vi "main_ui.vi"() -> ()   [LabVIEW 2014]
uses:
  <vilib>/Utility/miscctls.llb/LVPointDoubleTypeDef.ctl
  <vilib>/Analysis/1siggen.llb/Ramp Pattern by Samples.vi
  src/GLOBAL_VAR.vi
  <vilib>/Analysis/NI_AALBase.lvlib
panel:
  out "Laser power [mW]":dbl caption="Power" format="%.3f"
  in  "laser_on-off":bool caption="Laser"
  in  "T1_open":bool caption="Open T1"
  in  "esr_start":bool caption="Open ESR"
  in  "stop":bool
  in  "scan_start":bool
  in  "live-scan":bool
  out "ESR_stack":dbl[][](graph)
  out "X":dbl caption="X Rel" format="%.3f"
  out "Y":dbl caption="Y Rel" format="%.3f"
  out "XY Graph 2":cluster{"Value":dbl[], "Ramp Pattern":dbl[]}(graph)={"Value"=[-75.0, -71.93877551020408, -68.87755102040816, -65.81632653061224, -62.755102040816325, -59.69387755102041, -56.63265306122449, -53.57142857142857, -50.51020408163265, -47.44897959183673, -44.38775510204081, -41.3265306122449, -38.26530612244898, -35.204081632653065, -32.142857142857146, -29.081632653061227, -26.02040816326531, -22.95918367346939, -19.89795918367347, -16.836734693877553, -13.775510204081634, -10.714285714285722, -7.653061224489804, -4.591836734693885, -1.5306122448979664, 1.5306122448979522, 4.591836734693871, 7.6530612244897895, 10.714285714285708, 13.775510204081627, 16.836734693877546, 19.897959183673464, 22.959183673469383, 26.0204081632653, 29.08163265306122, 32.14285714285714, 35.20408163265306, 38.265306122448976, 41.326530612244895, 44.38775510204081, 47.44897959183673, 50.51020408163265, 53.571428571428555, 56.63265306122449, 59.69387755102039, 62.755102040816325, 65.81632653061223, 68.87755102040816, 71.93877551020407, 75.0], "Ramp Pattern"=[0.0, 0.0, 0.0, 0.0, 0.0, 0.0, 0.0, 0.0, 0.0, 0.0, 0.0, 0.0, 0.0, 0.0, 0.0, 0.0, 0.0, 0.0, 0.0, 0.0, 0.0, 0.0, 0.0, 0.0, 0.0, 0.0, 0.0, 0.0, 0.0, 0.0, 0.0, 0.0, 0.0, 0.0, 0.0, 0.0, 0.0, 0.0, 0.0, 0.0, 0.0, 0.0, 0.0, 0.0, 0.0, 0.0, 0.0, 0.0, 0.0, 0.0]}
  out "XY Graph":cluster{"Value":dbl[], "Ramp Pattern":dbl[]}(graph)={"Value"=[0.0, 0.0, 0.0, 0.0, 0.0, 0.0, 0.0, 0.0, 0.0, 0.0, 0.0, 0.0, 0.0, 0.0, 0.0, 0.0, 0.0, 0.0, 0.0, 0.0, 0.0, 0.0, 0.0, 0.0, 0.0, 0.0, 0.0, 0.0, 0.0, 0.0, 0.0, 0.0, 0.0, 0.0, 0.0, 0.0, 0.0, 0.0, 0.0, 0.0, 0.0, 0.0, 0.0, 0.0, 0.0, 0.0, 0.0, 0.0, 0.0, 0.0], "Ramp Pattern"=[-75.0, -71.93877551020408, -68.87755102040816, -65.81632653061224, -62.755102040816325, -59.69387755102041, -56.63265306122449, -53.57142857142857, -50.51020408163265, -47.44897959183673, -44.38775510204081, -41.3265306122449, -38.26530612244898, -35.204081632653065, -32.142857142857146, -29.081632653061227, -26.02040816326531, -22.95918367346939, -19.89795918367347, -16.836734693877553, -13.775510204081634, -10.714285714285722, -7.653061224489804, -4.591836734693885, -1.5306122448979664, 1.5306122448979522, 4.591836734693871, 7.6530612244897895, 10.714285714285708, 13.775510204081627, 16.836734693877546, 19.897959183673464, 22.959183673469383, 26.0204081632653, 29.08163265306122, 32.14285714285714, 35.20408163265306, 38.265306122448976, 41.326530612244895, 44.38775510204081, 47.44897959183673, 50.51020408163265, 53.571428571428555, 56.63265306122449, 59.69387755102039, 62.755102040816325, 65.81632653061223, 68.87755102040816, 71.93877551020407, 75.0]}
  out "scan_image":dbl[][](graph)
  out "wavechart_01":dbl(graph)
  in  "Tab Control":T1(tab)
  in  "counting_start":bool
  out "counts":dbl format="%.3e"
  in  "counts_dwell_time":dbl=30.0 caption="Dwell time [ms] :" min=0.0
  in  "pos-zero":bool caption="Blank Button"
  in  "scan_direction":enum32{"0", "1"}(radio)=enum."1" caption="Scan direction:"
  in  "frame_size_x_px":i32=100 caption="image_size_x"
  out "frame_size_y_px":i32=100 caption="image_size_y"
  out "pixel_size_z_um":dbl format="%#_3g"
  out "pixel_size_x_um":dbl=1.5 format="%#_3g"
  out "pixel_size_y_um":dbl=1.5 format="%#_3g"
  in  "pixel_dwell_ms":dbl=1.0 caption="Dwell time:"
  out "time_frame_s":dbl=10.0 caption="Time per frame:"
  in  "cursor-reset":bool caption="Blank Button"
  in  "pos-start_y":dbl caption="Y:" format="%#.3g"
  in  "pos-start_x":dbl caption="X:" format="%#.3f"
  in  "pos-start_cursor":bool caption="Blank Button"
  in  "pos_start":enum32{"bottom-left", "center"}(radio)=enum."center"
  in  "image_size_x_um":dbl=150.0 caption="X:"
  out "image_size_y_um":dbl=150.0 caption="Y:"
  in  "pos_z":dbl(slide) caption="Z:" scale=45.0..55.0
  in  "focus_z":dbl caption="Focus :" min=0.0 max=100.0 step=0.001 format="%.3f"
  in  "focus_dwell_ms":dbl=100.0 caption="Dwell :"
  in  "focus_q_steps":i32=100 caption="Steps :"
  in  "focus_z_end":dbl=100.0 caption="End :"
  in  "focus_z_start":dbl caption="Start :"
  in  "focus_start":bool
  out "timeseries-rem_time":string caption="Remaining time :"
  in  "timeseries-autofocus":enum16{"No autofocus", "Max x-y", "Center"}(ring) caption="Autofocus :"
  out "timeseries-current_image":dbl caption="Current scan :" format="%#.3f"
  out "timeseries-total_images":dbl=1.0 caption="Total scans :" format="%#.3f"
  in  "timeseries-start":bool
  in  "timeseries-period":dbl caption="Period :" format="%#.3f"
  in  "timeseries-stopdate":timestamp=timestamp(3557915984.536238 s since 1904-01-01) caption="Stop at :" format="%<%X\n%x>T"
  out "timeseries-next_scan":timestamp caption="Next scan at :" format="%<%X\n%x>T"
  in  "Z-stack_enable":bool
  in  "z-stack_slices":i32=1 caption="Slices :" min=1 step=1
  out "z-stack_step_size":dbl caption="Step size :" format="%#.4f"
  in  "Z-stack_tabs":enum32{"From-To", "Centering"}(tab)
  in  "z-stack-set_to":bool
  in  "z-stack-set_from":bool
  in  "z-stack_to":dbl=100.0 caption="To :"
  in  "z-stack_from":dbl caption="From :"
  in  "z-stack-set_center":bool
  in  "z-stack_size":dbl=10.0 caption="Size :"
  in  "z-stack_center":dbl=5.0 caption="Center :"
  in  "z-stack_pos":i32(slide)=1 caption="Z slice :" min=1 step=1 scale=1.0..1.1
  in  "current_z":dbl caption="Z :" min=0.0 max=100.0 step=0.0001 format="%.4f"
  in  "current_y":dbl caption="Y :" min=-10.0 max=10.0 step=0.0001 format="%.4f"
  in  "current_x":dbl caption="X :" min=-10.0 max=10.0 step=0.0001 format="%.4f"
  in  "recenter":bool caption="Laser"
  in  "continious_recenter":bool
  in  "parameters_xy-scan":T2={"image_size_xy_um"=0.5, "frame_size_xy_px"=20, "dwell_time_ms"=1.0}
  in  "parameters_z-scan":T3={"dwell_time_ms"=10.0, "q_steps"=20, "span_um"=2.0, "refocus"=TRUE}
  out "particle_lost":bool
  in  "XY Max focus?":bool
  in  "X Zero":dbl format="%.3f"
  in  "Y Zero":dbl format="%.3f"
  in  "X Rel":dbl format="%.3f"
  in  "Y Rel":dbl format="%.3f"
  out "upos-xy_control":cluster{"X":dbl, "Y":dbl}[](graph)
  in  "upos-stop":bool
  in  "upos-x":dbl caption="X:" min=0.0 max=8.0 format="%.3f"
  in  "upos-y":dbl caption="Y:" min=0.0 max=8.0 format="%.3f"
  out "upos-cpos_y":dbl format="%#.3f"
  out "upos-cpos_x":dbl format="%#.3f"
  out "upos-state_x":u32 caption="X:"
  out "upos-state_y":u32 caption="Y:"
  in  "tiles-overlap":dbl=10.0 caption="Overlap :"
  out "tile_progress":u8(slide) caption="Progress :" scale=0.0..100.0
  out "tile_remaining_tiles":dbl caption="Remaining\ntiles :"
  out "tile_remaining_time":dbl caption="Remaining\ntime :"
  in  "tile-scan_start":bool
  in  "tile_tiles-size":enum32{"tiles", "size"}(radio)=enum."size"
  out "tile_q-tiles_y":dbl=1.0 caption="Y :"
  in  "tile_q-tiles_x":dbl=1.0 caption="X :"
  out "tile_size_y_um":dbl=10.0 caption="Y:"
  in  "tile_size_x_um":dbl=10.0 caption="Size :"
  in  "tile_start_y_mm":dbl caption="Y:" format="%#.3g"
  in  "tile_start_x_mm":dbl caption="X:" format="%#.3f"
  out "esr_generator_ok":bool caption="Generator\nstatus :"
  out "esr_current_run":i32 caption="Run :"
  in  "esr_out_enable":bool caption="Output on/off :"
  out "esr_power_led":bool
  out "esr_remain":i32 caption="Remain :"
  in  "esr_repetitions":i32=1 caption="Repetitions" min=1 max=1000 step=1
  in  "esr_dwell_time":ext=0.09999999974525053 caption="Dwell Time :" format="%.3f"
  in  "esr_step_size":ext=2500000.0 caption="Step size :" format="%.2p"
  in  "esr_freq_stop":ext=3000000000.0 caption="Freq Stop :" format="%.2p"
  in  "esr_freq_start":ext=2800000000.0 caption="Freq Start :" format="%.2p"
  out "esr_total_time":ext=8120.249980327117 caption="Total time :"
  in  "esr_power":ext=5.999999061226845 caption="Power :" format="%.2f"
  in  "live_scan_direction":enum32{"0", "1"}(radio)=enum."1" caption="Scan direction:"
  in  "live_frame_size_x_px":i32=50 caption="image_size_x"
  in  "live_pixel_dwell_ms":dbl=0.5 caption="Dwell time:"
  in  "objective":u16(ring)=1 items=["Raw scale (volts)", "UPlanSApo 100x / 1,40 Oil", "UPlanSApo 40X / 0,95 Air"]
  in  "file_save":bool
  in  "file_autosave":bool
  in  "file_path":path caption="Folder :"
  in  "file_name":string caption="Name :"
  in  "save_tiff":bool
  in  "save_txt":bool
  # "Relative cursor position [um]"
  # "Scanning area [mm]"
  # "Size:"
  # "x"
  # "Position:"
  # "Acquisition"
  # "Frame size:"
  # "x"
  # "px"
  # "ms"
  # "Pixel size [mm] :"
  # "x"
  # "x"
  # "Seconds"
  # "Manual focus [mm]"
  # "Auto-focus [mm]"
  # "ms"
  # "Photon counting"
  # "Time series"
  # "[s]"
  # "Z stack [mm]"
  # "Set position [mm]"
  # "Refocus"
  # "Positioners (xy motors)"
  # "Absolute"
  # "Zeros"
  # "Relative"
  # "Status"
  # "State :"
  # "Position :"
  # "Tiles scan"
  # "Start position [mm]:"
  # "mm"
  # "mm"
  # "mm"
  # "min"
  # "Sweep"
  # "Hz"
  # "Hz"
  # "Hz"
  # "ms"
  # "dBm"
  # "s"
  # "Objective"
  # "Live scan"
  # "Frame size:"
  # "px"
  # "ms"
  # "Save"
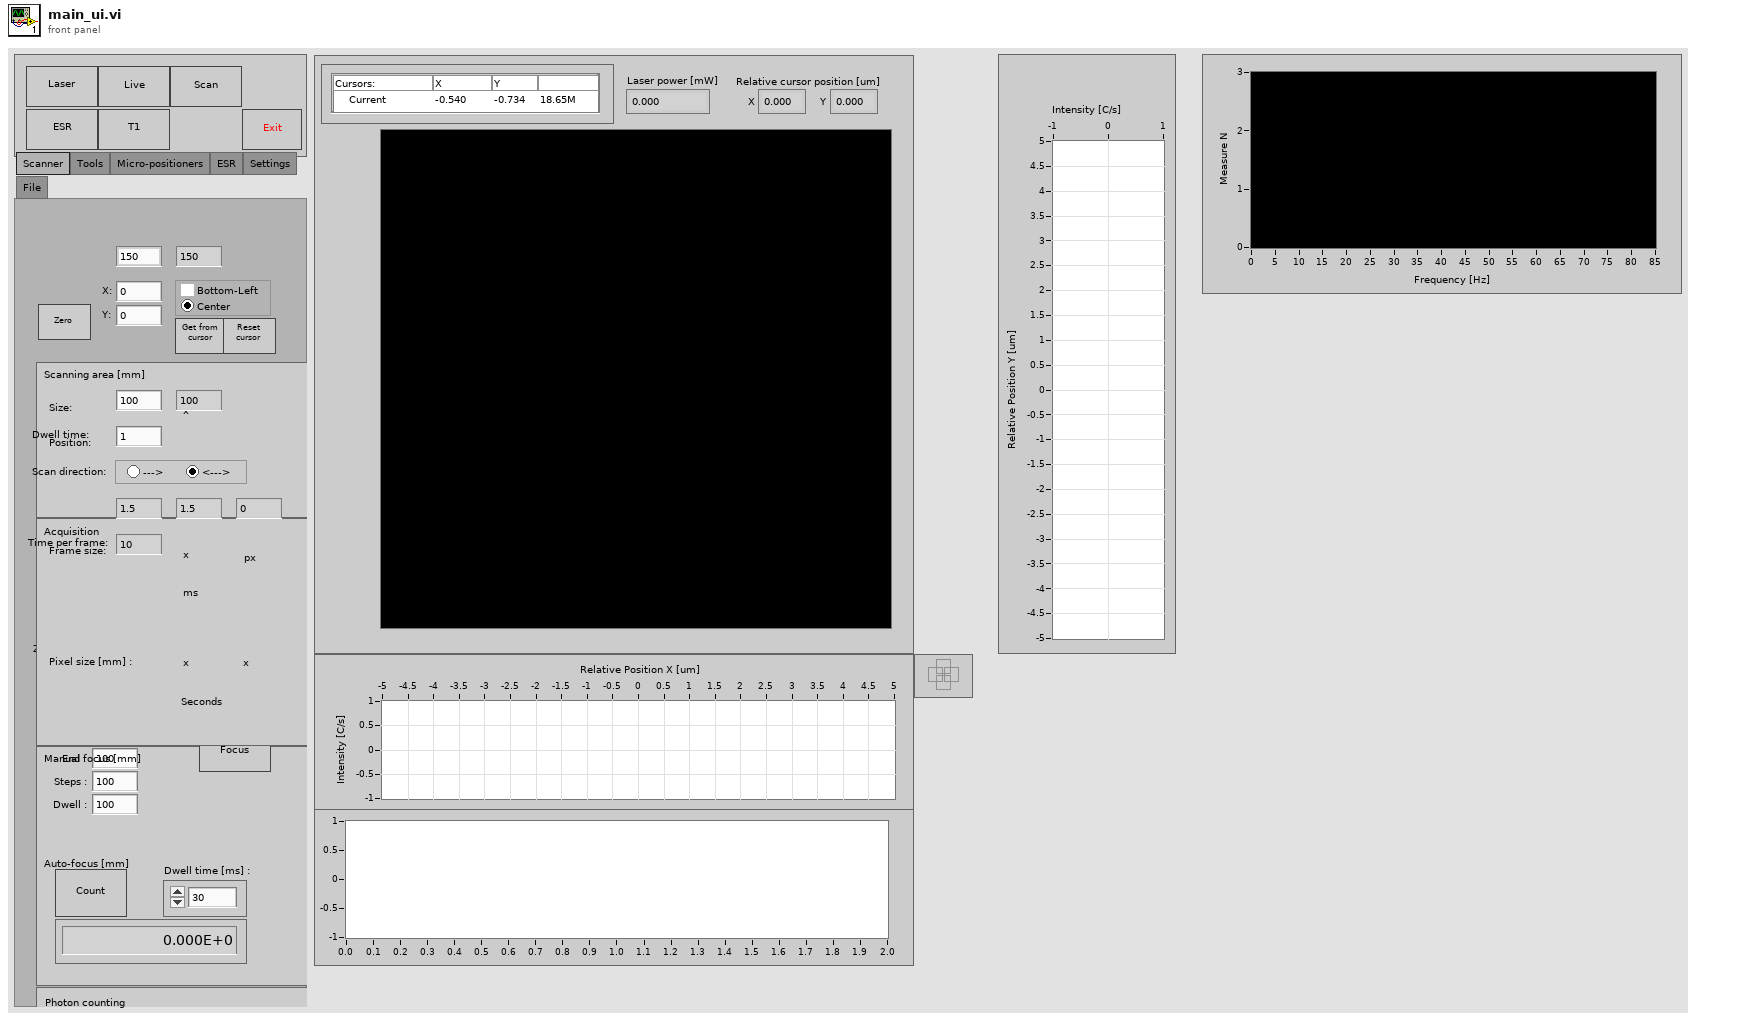
[diagram p1: front panel]
types:
  T1 = enum32{"Scanner", "Tools", "Micro-positioners", "ESR", "Settings", "File"}
  T2 = cluster{"image_size_xy_um":dbl, "frame_size_xy_px":u32, "dwell_time_ms":dbl}
  T3 = cluster{"dwell_time_ms":dbl, "q_steps":u32, "span_um":dbl, "refocus":bool}
  T4 = cluster{"status_x":dbl, "status_y":dbl, "status_z":dbl, "pos_x":dbl, "pos_y":dbl, "pos_z":dbl}
  T5 = cluster{enum16{"standby", "domove", "dostop", "exit", "status"}, dbl, dbl, dbl}
  T6 = typedef "LVPointDoubleTypeDef.ctl" = cluster{"X":dbl, "Y":dbl}
  T7 = enum8{"Enabled", "Disabled", "Disabled and Grayed Out"}
  T8 = cluster{"overlap":dbl, "pos-xy_start":cluster{"pos-x_start":dbl, "pos-y_start":dbl}, "pos-xy_end":cluster{"pos-x_end":dbl, "pos-y_end":dbl}, "pos-xy_ref":cluster{"pos-x_start":dbl, "pos-y_start":dbl}}
  T9 = cluster{"z_start":dbl, "z_end":dbl, "q_steps":i32, "dwell_time_ms":dbl}
  T10 = cluster{"image_size":dbl, "image_xy_start":cluster{"image-x_start":dbl, "image-y_start":dbl}, "pixel_dwell_ms":dbl, "frame_size_x_px":i32, "scan_direction":enum32{"0", "1"}, "pos_start":enum32{"bottom-left", "center"}}
  T11 = cluster{"nano-position_X_um":sgl, "nano-position_Y_um":sgl, "nano-position Z_um":sgl}
  T12 = enum16{"Standby", "doScan", "doCount", "doFocus", "doLiveScan", "do3DScan"}
  T13 = enum16{"Standby", "doScan", "doCount", "doFocus", "doLiveScan"}
  T14 = enum16{"Standby", "doScan", "doCount", "doFocus", "doLiveScan", "do3DScan", "changeZslice", "doESR", "doTileScan", "doStartPos", "doTimeseries"}
  T15 = enum16{"Standby", "doScan", "doCount", "doFocus"}
  T16 = enum16{"Standby", "doScan", "doCount", "doFocus", "doLiveScan", "do3DScan", "changeZslice", "doESR", "doTileScan", "doStartPos", "doTimeseries", "saveImage", "doT1", "doRecenter"}
  T17 = enum16{"Standby", "doScan", "doCount", "doFocus", "doLiveScan", "do3DScan", "changeZslice"}
  T18 = enum16{"Standby", "doScan", "doCount", "doFocus", "doLiveScan", "do3DScan", "changeZslice", "doESR"}
  T19 = enum16{"Standby", "doScan", "doCount", "doFocus", "doLiveScan", "do3DScan", "changeZslice", "doESR", "doTileScan"}
  T20 = enum16{"standby", "domove", "dostop", "exit", "status"}
  T21 = enum16{"Standby", "doScan", "doCount", "doFocus", "doLiveScan", "do3DScan", "changeZslice", "doESR", "doTileScan", "doStartPos", "doTimeseries", "saveImage", "doT1"}
  T22 = enum16{"Standby", "doScan", "doCount", "doFocus", "doLiveScan", "do3DScan", "changeZslice", "doESR", "doTileScan", "doStartPos", "doTimeseries", "saveImage"}
  T23 = cluster{enum16{"standby", "domove", "dostop", "exit", "status"}, "Value":dbl, "Value":dbl, "Value":dbl}
  T24 = cluster{enum16{"standby", "domove", "dostop", "exit", "status"}, dbl, dbl, "Value":dbl}
  T25 = cluster{enum16{"standby", "domove", "dostop"}, "X":dbl, "Y":dbl, dbl}
  T26 = cluster{enum16{"standby", "domove", "dostop", "exit"}, "upos-x":dbl, "upos-y":dbl, dbl}
  T27 = cluster{enum16{"standby", "domove", "dostop", "exit"}, dbl, dbl, dbl}
  T28 = cluster{"pos-start_x":dbl, "pos-start_y":dbl, "focus_z":dbl}
  T29 = cluster{"file_path":path, "file_name":string, "image":dbl[][][], "image_size_xy":cluster{"image_size_x_um":sgl, "image_size_y_um":sgl}, "pixel_dwell_time_ms":sgl, "Laser_power_mW":sgl, "pixel_size":dbl, "tile_ij":cluster{"tile_i":i32, "tile_j":i32}, "Objective":string, "ColorMarkers":cluster{dbl, u32}[], "timestamp":timestamp, "micro-position-xyz":cluster{"micro-position_x_mm":sgl, "micro-position_y_mm":sgl, "micro-position_z_mm":sgl}, "zero_xyz":cluster{"zero_x_mm":dbl, "zero_y_mm":dbl, "zero_z_mm":dbl}, "nano-position-xyz":cluster{"nano-position_x_V":sgl, "nano-position_y_V":sgl, "nano-position_z_V":sgl}, "Kxyz":cluster{"Kx_V/um":sgl, "Ky_V/um":sgl, "Kz_V/um":sgl}}
  T30 = cluster{"image_size_x_um":dbl, "image_size_x_um":dbl}
  T31 = cluster{"esr_repetitions":i32, "esr_power":ext, "esr_freq_start":ext, "esr_freq_stop":ext, "esr_step_size":ext, "esr_dwell_time":ext}
  T32 = cluster{"Cursor.Cursor X":dbl, "Cursor.Cursor Y":dbl, "focus_z":dbl}
  T33 = cluster{"tile_start_x_mm":dbl, "tile_start_y_mm":dbl}
  T34 = cluster{"Value":dbl, "Value":dbl, "Value":i32, "Value":bool}
  T35 = cluster{"timeseries-current_image":refnum<vi>, "scan_image":refnum<vi>, "timeseries-start":refnum<vi>, "timeseries-next_scan":refnum<vi>, "timeseries-rem_time":refnum<vi>}
  T36 = cluster{"X Zero":dbl, "Y Zero":dbl, "upos-y":dbl}
  T37 = cluster{"Cursor.Cursor X":dbl, "Cursor.Cursor Y":dbl, "Value":dbl}
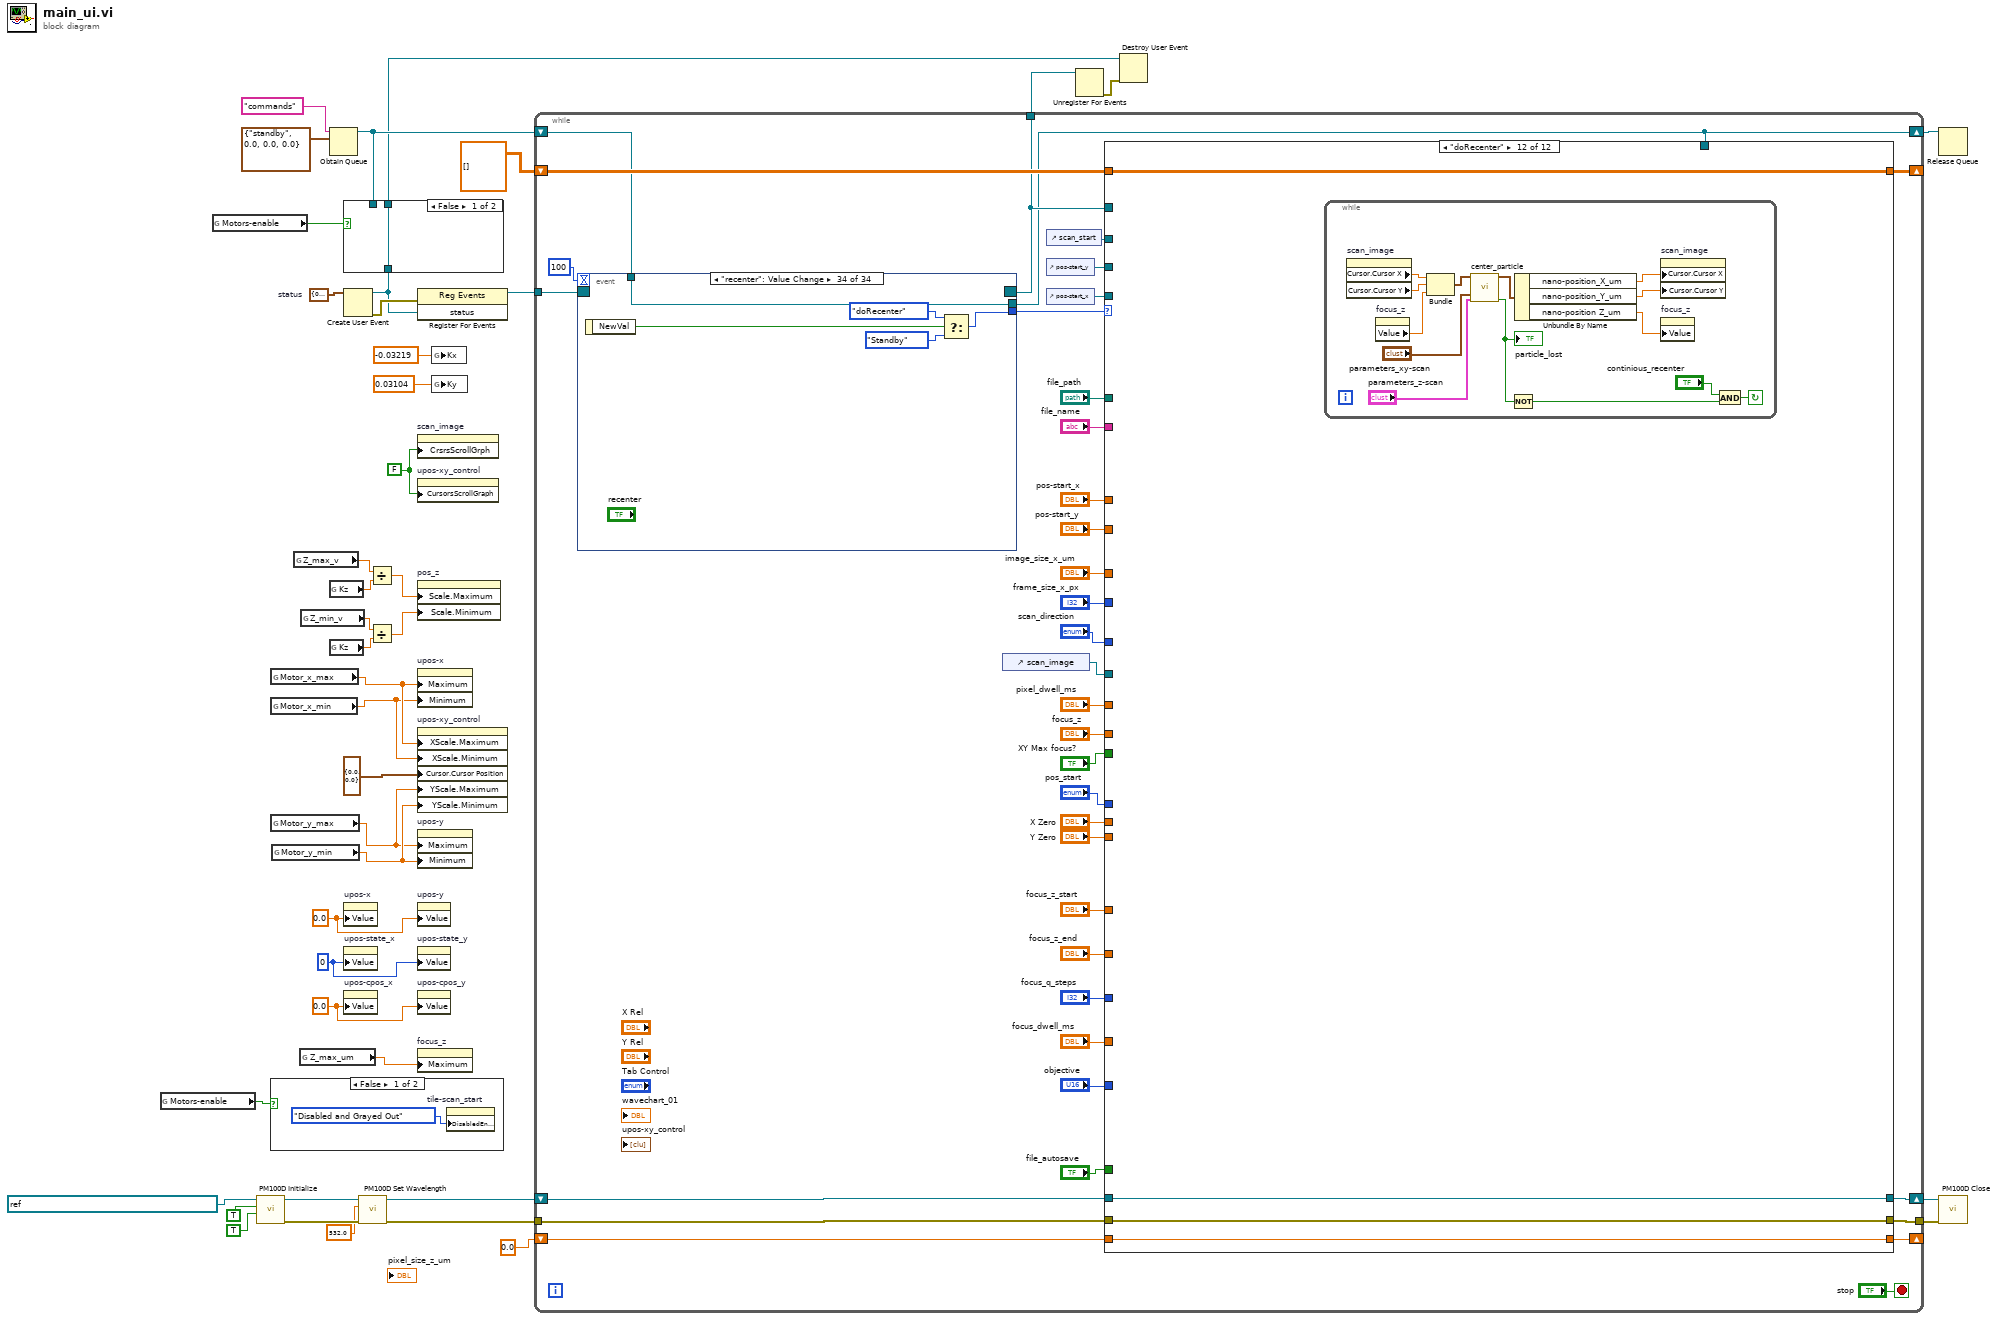
[diagram p0: block diagram]
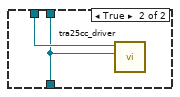
[diagram p2: hidden frame]
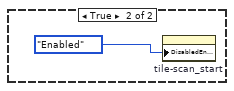
[diagram p3: hidden frame]
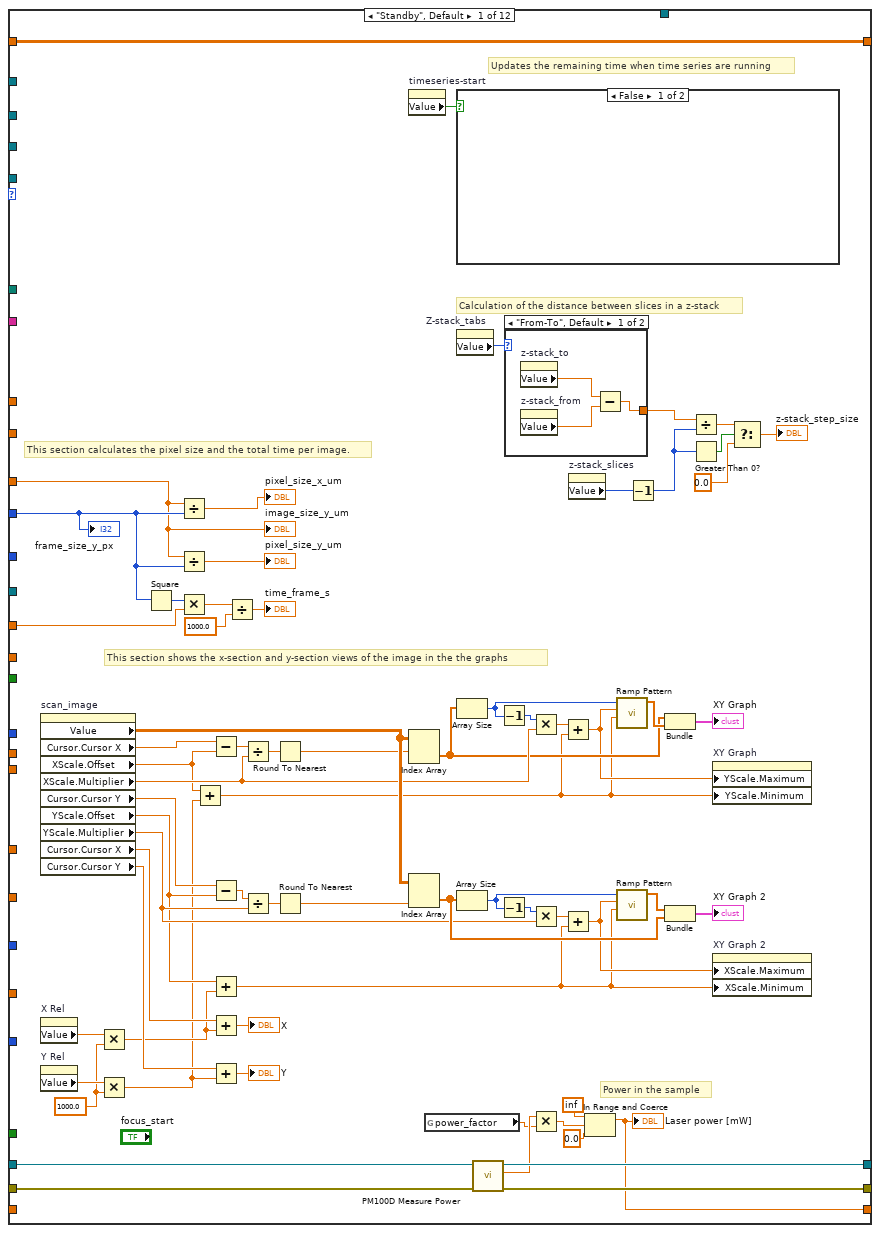
[diagram p4: hidden frame]
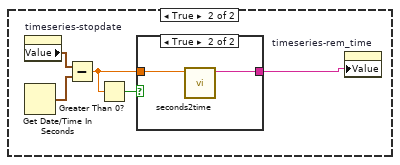
[diagram p5: hidden frame]
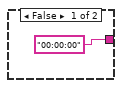
[diagram p6: hidden frame]
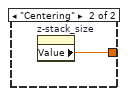
[diagram p7: hidden frame]
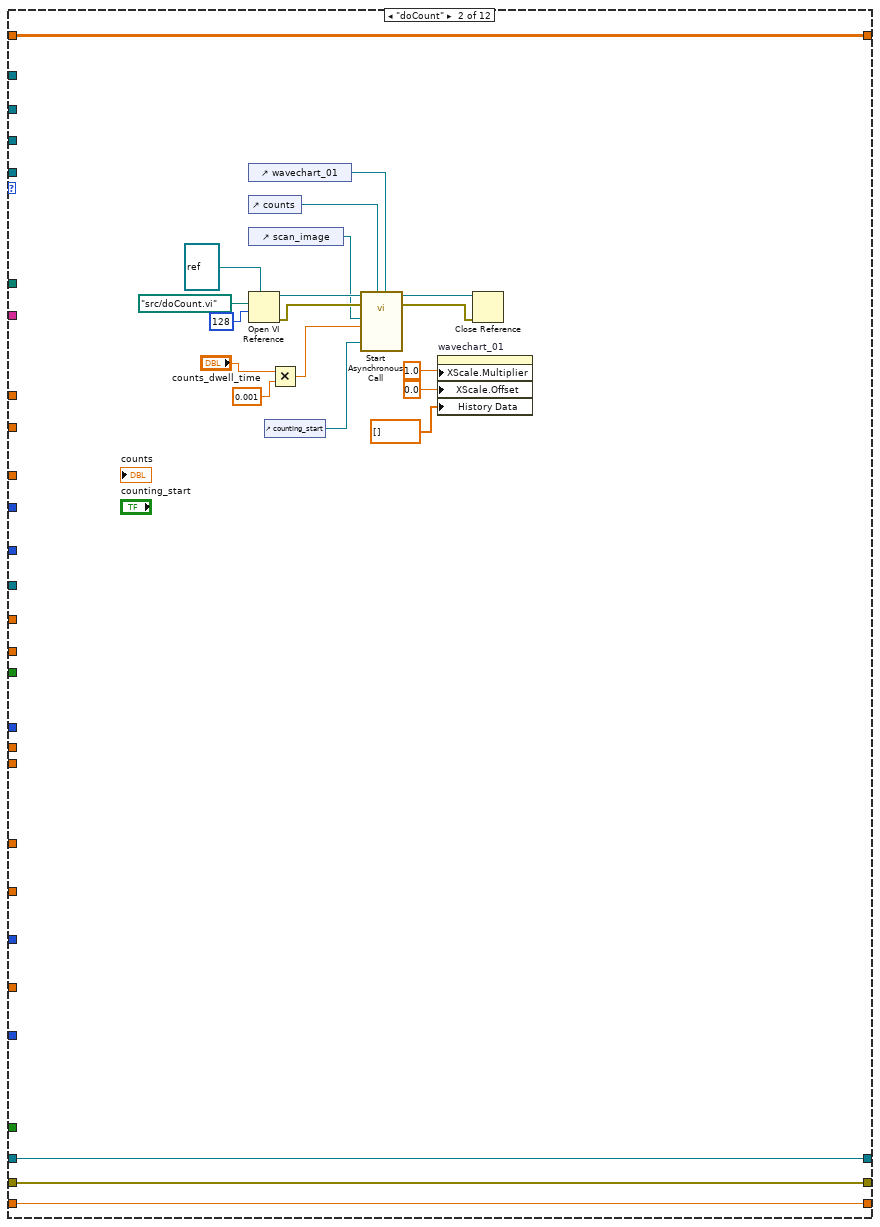
[diagram p8: hidden frame]
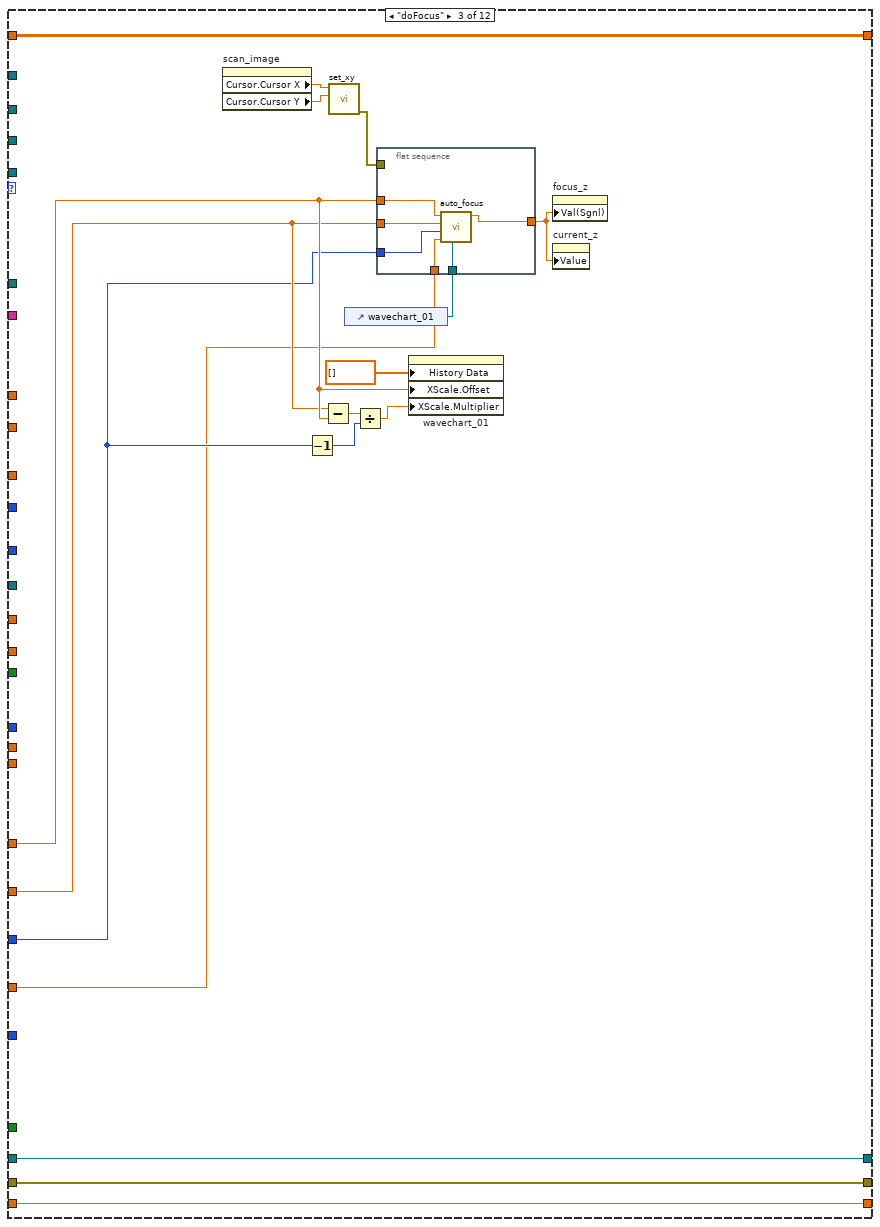
[diagram p9: hidden frame]
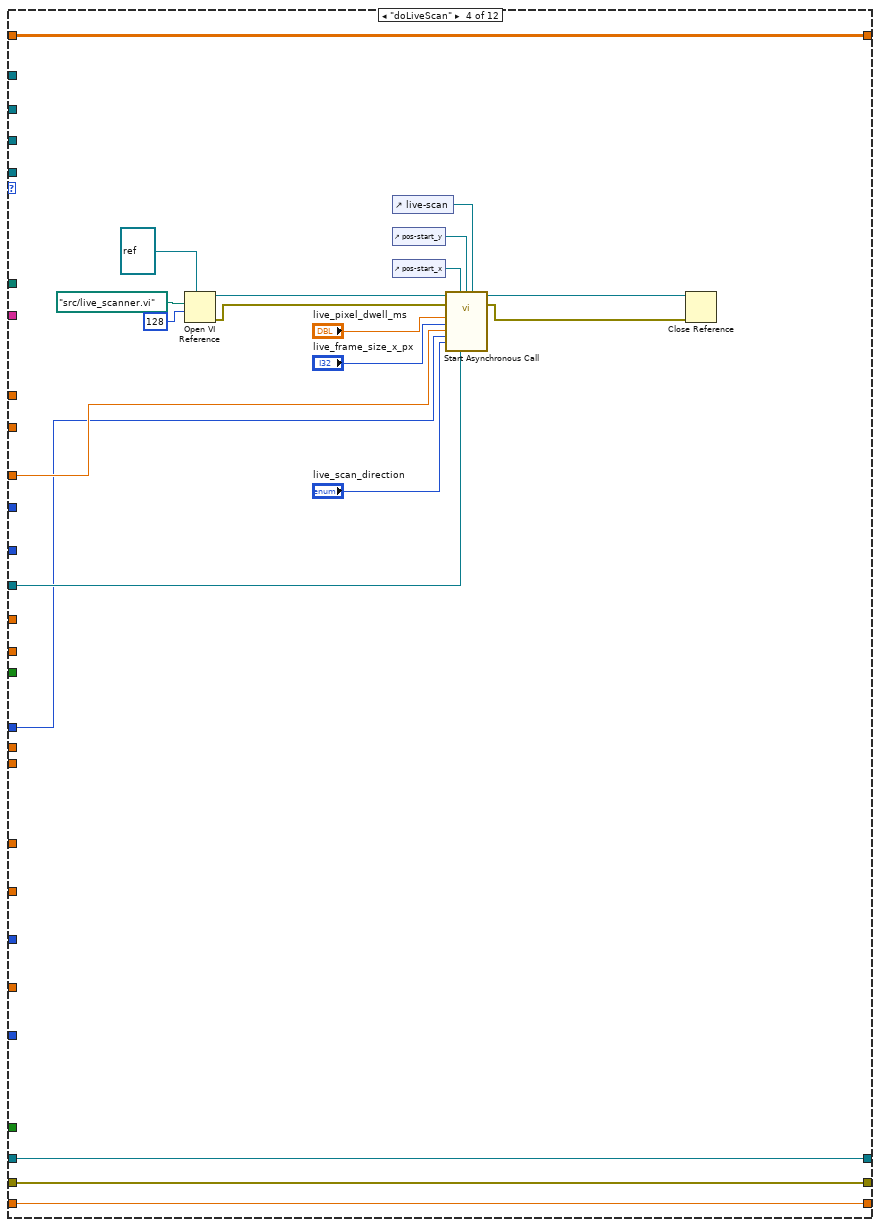
[diagram p10: hidden frame]
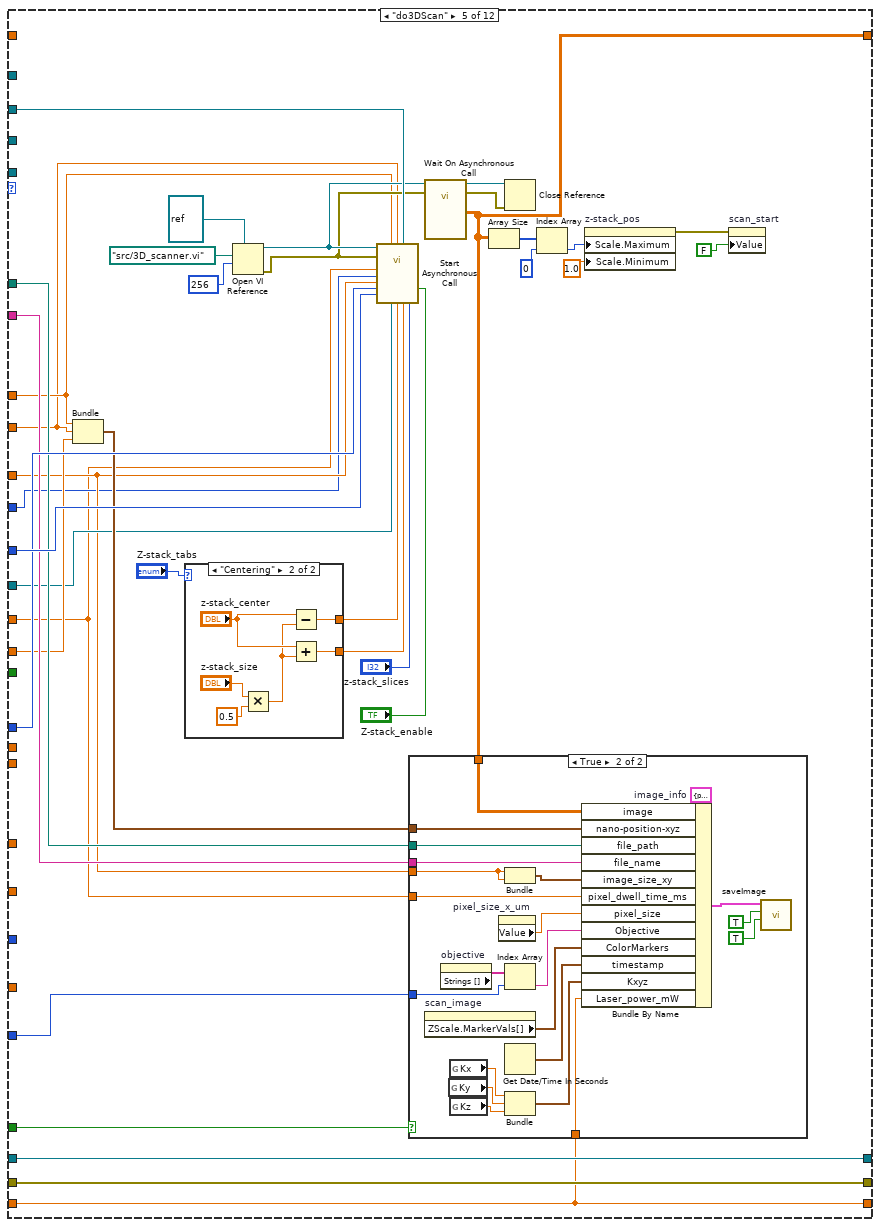
[diagram p11: hidden frame]
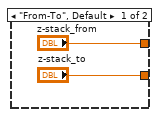
[diagram p13: hidden frame]
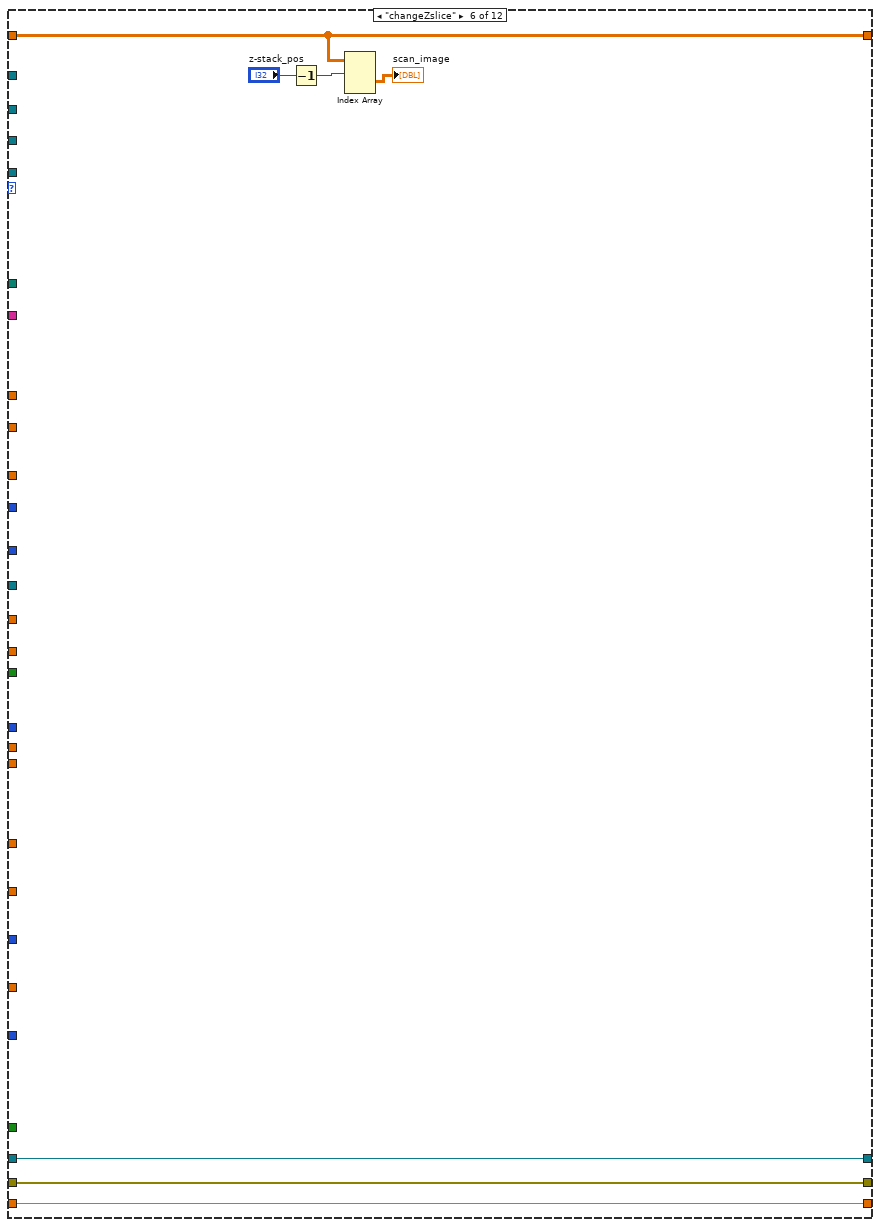
[diagram p14: hidden frame]
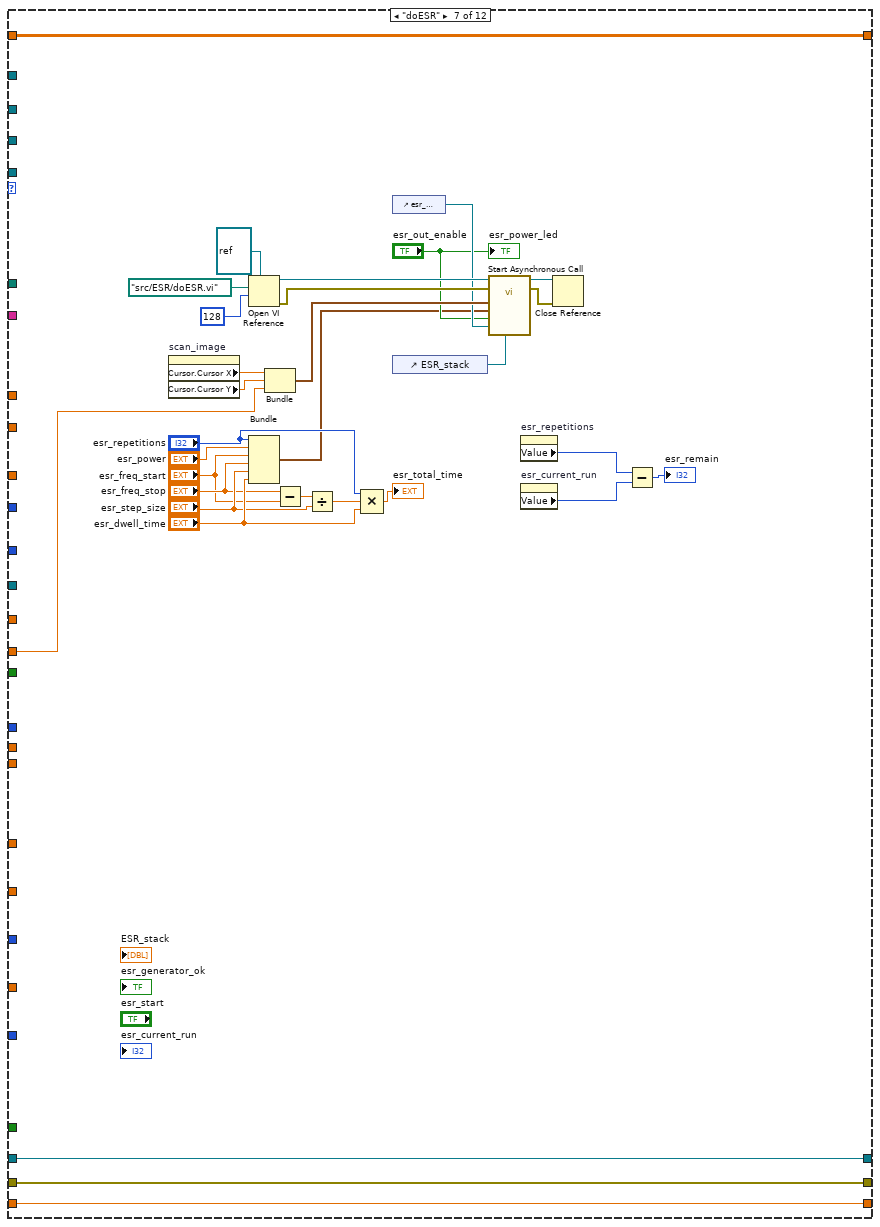
[diagram p15: hidden frame]
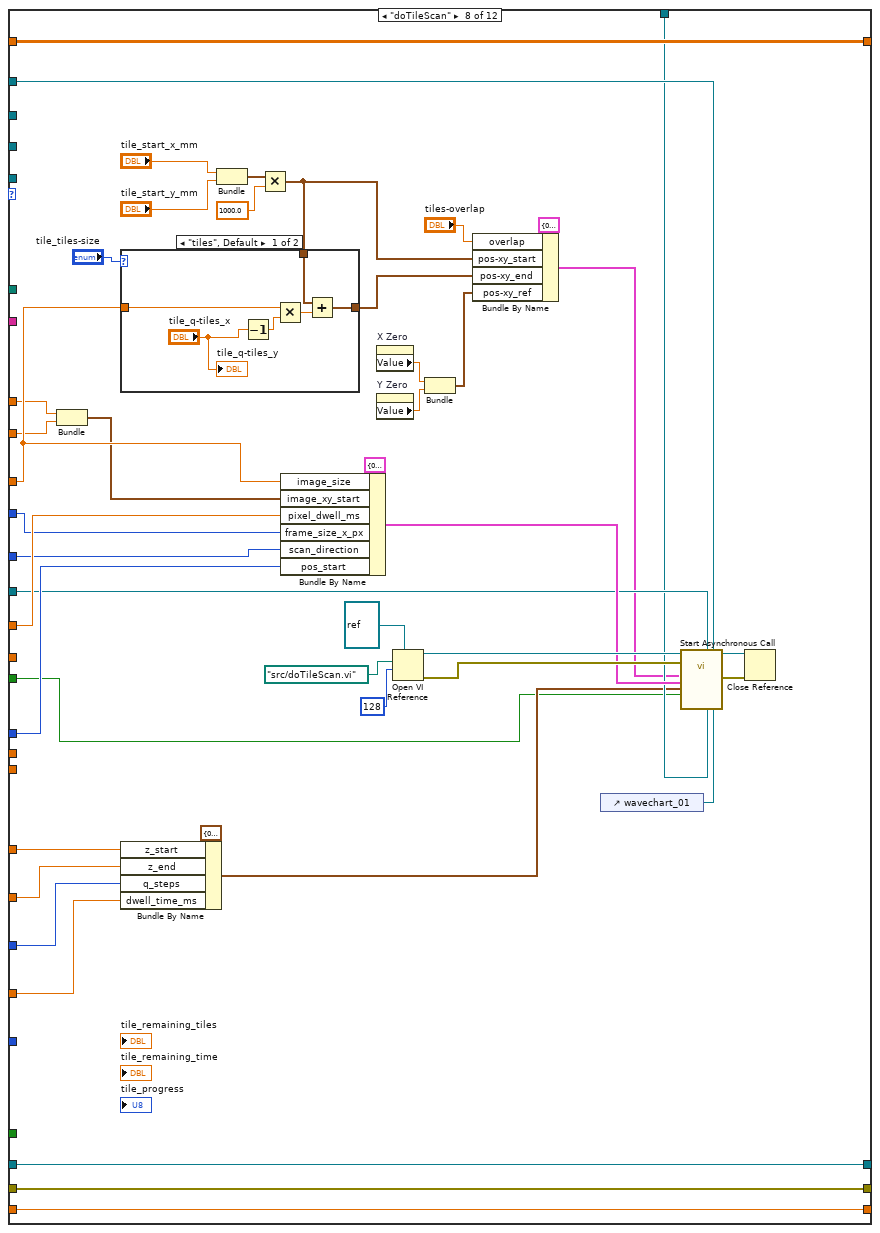
[diagram p16: hidden frame]
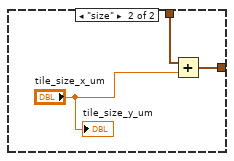
[diagram p17: hidden frame]
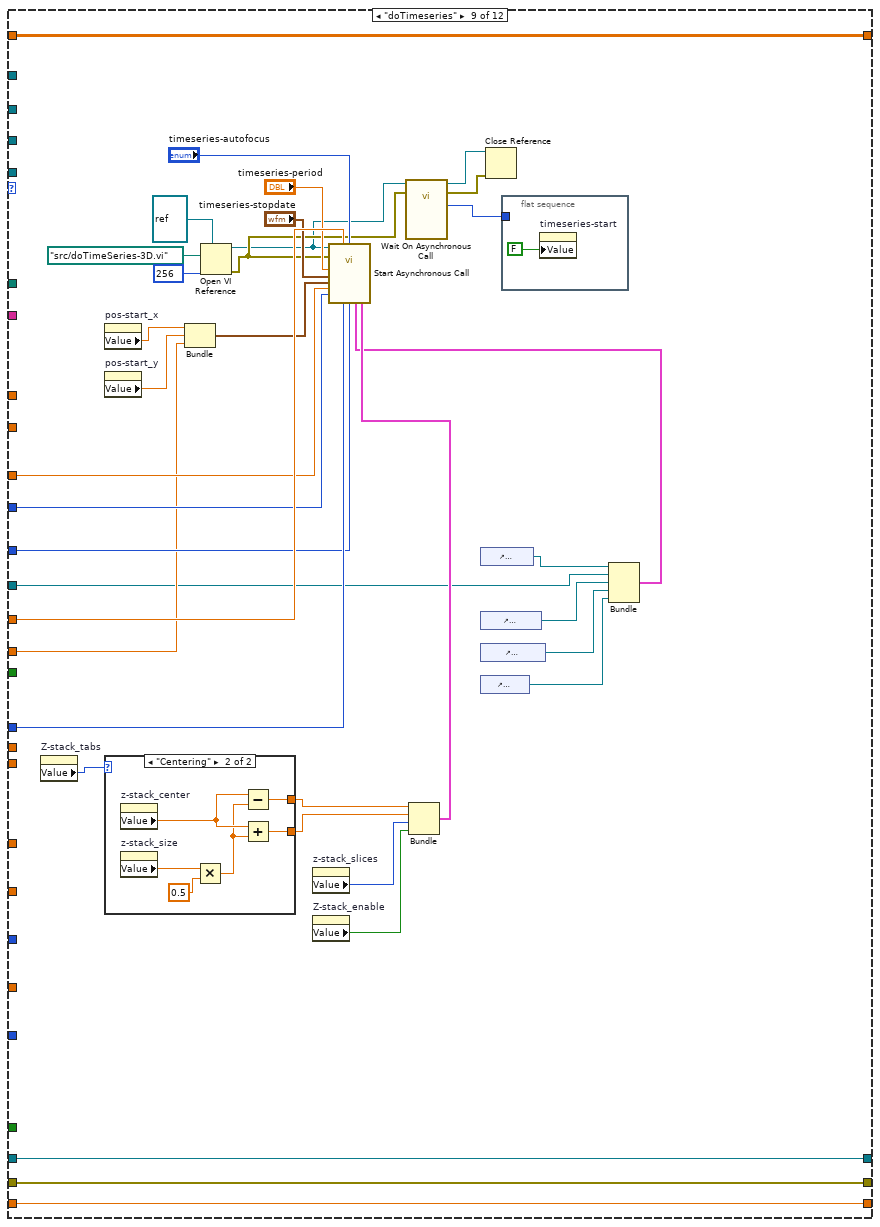
[diagram p18: hidden frame]
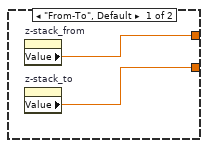
[diagram p19: hidden frame]
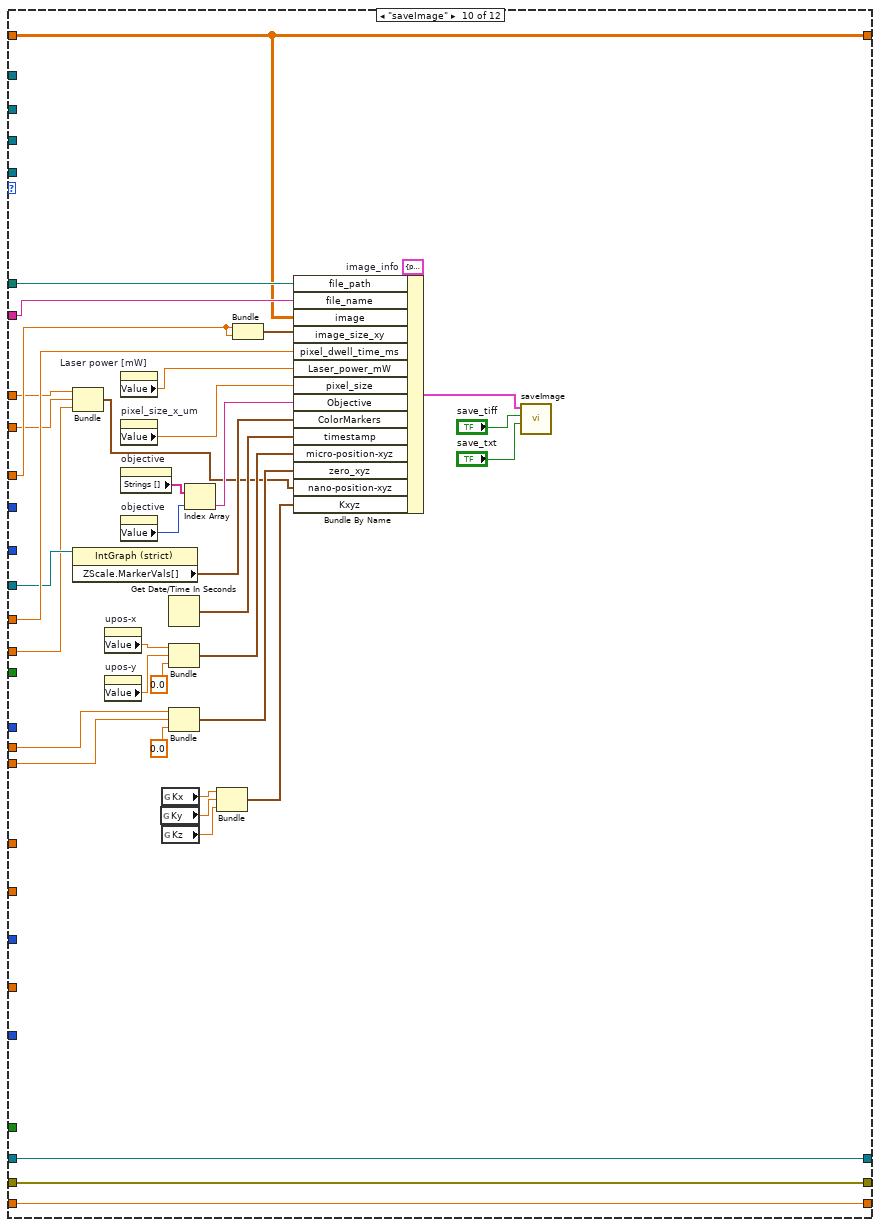
[diagram p20: hidden frame]
diagram:
  w24 = T4 {"status_x"=0.0, "status_y"=0.0, "status_z"=0.0, "pos_x"=0.0, "pos_y"=0.0, "pos_z"=0.0}  # status
  w28 = 0.0 ("upos-cpos_x")
  w29 = u32 0 ("upos-state_x")
  w30 = 0.0 ("upos-x")
  w36 = FALSE ("Cursors Scroll Graph")
  n1 = global read "GLOBAL_VAR.vi" "Motors-enable"() -> (w27:bool)
  n2 = global read "GLOBAL_VAR.vi" "Motors-enable"() -> (w17:bool)
  n3 = call <instrlib>:"PM100D Initialize.vi"("Reset Device (Reset Device)"=TRUE ("ID Query (Do Query)"), "ID Query (Do Query)"=TRUE, "resource name"=refnum<visa-resource-name> "USB0::0x1313::0x8072::P2008372::INSTR") -> ("error out"=w5:errorcluster, "instrument handle out"=w4:refnum<visa-resource-name>)  [unwired: 7 in]
  n4 = global read "GLOBAL_VAR.vi" "Motor_x_max"() -> (w35:dbl)
  n5 = global read "GLOBAL_VAR.vi" "Motor_x_min"() -> (w34:dbl)
  n6 = global read "GLOBAL_VAR.vi" "Motor_y_max"() -> (w32:dbl)
  n7 = case shown="False" w27 {
    frame False {
      n8 = property on="tile-scan_start" class="Bool (strict)"("DisabledEnum"=T7."Disabled and Grayed Out" ("Disabled")) -> ()  [unwired: 2 in, 2 out]
    }
    frame True {
      n9 = property on="tile-scan_start" class="Bool (strict)"("DisabledEnum"=T7."Enabled" ("Disabled")) -> ()  [unwired: 2 in, 2 out]
    }
  }
  n10 = global read "GLOBAL_VAR.vi" "Motor_y_min"() -> (w33:dbl)
  n11 = global read "GLOBAL_VAR.vi" "Z_max_v"() -> (w43:dbl)
  n12 = global read "GLOBAL_VAR.vi" "Z_max_um"() -> (w12:dbl)
  n13 = global read "GLOBAL_VAR.vi" "Z_min_v"() -> (w40:dbl)
  n14 = Obtain Queue(name (unnamed)="commands", element data type=T5 {enum."standby", 0.0, 0.0, 0.0}) -> (queue out=w18:refnum<queue>)  [unwired: 3 in, 2 out]
  n15 = global read "GLOBAL_VAR.vi" "Kz"() -> (w42:dbl)
  n16 = global read "GLOBAL_VAR.vi" "Kz"() -> (w39:dbl)
  n17 = Create User Event(user event datatype=w24) -> (user event=w16:refnum<user-event>, error out=w23:errorcluster)  [unwired: 1 in]
  n18 = case shown="False" w17 {
    tunnel: w16 -> [w46 w47]
    tunnel: w18 -> [_ w48]
    tunnel: [w46 w47] -> w15
    frame False {
    }
    frame True {
      n19 = call "tra25cc_driver.vi"("user_event-status_in"=w47, "queue-commands"=w48) -> ()  [unwired: 9 in, 1 out]
    }
  }
  n20 = property on="upos-x" class="DigNum (strict)"("Value"=w30) -> ()  [unwired: 2 in, 2 out]
  n21 = property on="upos-state_x" class="DigNum (strict)"("Value"=w29) -> ()  [unwired: 2 in, 2 out]
  n22 = property on="upos-cpos_x" class="DigNum (strict)"("Value"=w28) -> ()  [unwired: 2 in, 2 out]
  n23 = call <instrlib>:"PM100D Set Wavelength.vi"("error in (no error)"=w5, "Wavelength (0.0)"=532.0, "instrument handle"=w4) -> ("error out"=w10:errorcluster, "instrument handle out"=w11:refnum<visa-resource-name>)  [unwired: 7 in]
  n24 = Divide(x=w43, y=w42) -> (x/y=w41:dbl)
  n25 = Divide(x=w40, y=w39) -> (x/y=w38:dbl)
  n26 = register-events(error in=w23, w16) -> (reference out=w22:refnum<event-registration>)  [unwired: 1 in, 1 out]
  n27 = property on="scan_image" class="IntGraph (strict)"("CrsrsScrollGrph"=w36) -> ()  [unwired: 2 in, 2 out]
  n28 = property on="upos-xy_control" class="XYGraph (strict)"("CursorsScrollGraph"=w36) -> ()  [unwired: 2 in, 2 out]
  n29 = property on="pos_z" class="Slide (strict)"("Scale.Maximum"=w41, "Scale.Minimum"=w38) -> ()  [unwired: 2 in, 2 out]
  n30 = property on="upos-x" class="DigNum (strict)"("Maximum"=w35, "Minimum"=w34) -> ()  [unwired: 2 in, 2 out]
  n31 = property on="upos-xy_control" class="XYGraph (strict)"("XScale.Maximum"=w35, "XScale.Minimum"=w34, "Cursor.Cursor Position"=T6 {"X"=0.0, "Y"=0.0}, "YScale.Maximum"=w32, "YScale.Minimum"=w33) -> ()  [unwired: 2 in, 2 out]
  n32 = property on="upos-y" class="DigNum (strict)"("Maximum"=w32, "Minimum"=w33) -> ()  [unwired: 2 in, 2 out]
  n33 = property on="upos-y" class="DigNum (strict)"("Value"=w30) -> ()  [unwired: 2 in, 2 out]
  n34 = property on="upos-state_y" class="DigNum (strict)"("Value"=w29) -> ()  [unwired: 2 in, 2 out]
  n35 = property on="upos-cpos_y" class="DigNum (strict)"("Value"=w28) -> ()  [unwired: 2 in, 2 out]
  n36 = property on="focus_z" class="DigNum (strict)"("Maximum"=w12) -> ()  [unwired: 2 in, 2 out]
  n37 = global write "GLOBAL_VAR.vi" "Kx"(-0.03219 ("Kx")) -> ()
  n38 = global write "GLOBAL_VAR.vi" "Ky"(0.03104 ("Kx")) -> ()
  n39 = while {
    shift-right: [w85] -> _
    shift-left: dbl[][][] [] ("image_out") -> [w84]
    tunnel: w22 -> [w74]
    tunnel: [w71] -> w21
    shift-right: [w70] -> w19
    shift-left: w18 -> [w72]
    tunnel: w10 -> [w61]
    tunnel: [w59] -> w9
    shift-right: [w52] -> _
    shift-left: 0.0 ("upper limit") -> [w51]
    shift-right: [w60] -> w8
    shift-left: w11 -> [w62]
    stop <- "stop" stop-if-true
    n40 = event shown="[33] \"recenter\": Value Change" {
      selector: w74 -> [_ _ _ _ _ _ _ _ _ _ _ _ _ _ _ _ _ _ _ _ _ _ _ _ _ _ _ _ _ _ _ _ _ _]
      dyn-events: [_ _ _ _ _ _ _ _ _ _ _ _ _ _ _ _ _ _ _ _ _ _ _ _ _ _ _ _ _ _ _ _ _ _] -> w71
      timeout: 100 -> [_ _ _ _ _ _ _ _ _ _ _ _ _ _ _ _ _ _ _ _ _ _ _ _ _ _ _ _ _ _ _ _ _ _]
      tunnel: [T12."Standby" w513 w518 w519 w526 T15."Standby" T13."Standby" T15."Standby" T13."Standby" T13."Standby" T13."Standby" T16."Standby" T12."Standby" T12."Standby" T12."Standby" T12."Standby" T17."changeZslice" T17."Standby" w593 w600 w605 T16."Standby" T16."doRecenter" T16."Standby" T16."Standby" T16."Standby" _ _ _ _ _ w704 w711 w713] -> w86
      tunnel: w72 -> [w507 w509 w514 w523 w524 w529 w533 w536 w550 w559 w562 w566 w569 w572 w575 w578 w583 w585 w589 w594 w601 w617 w626 w631 w645 w654 w662 w672 w677 w685 w700 w706 w707 w712]
      tunnel: [w507 w509 w514 w523 w524 w529 w533 w536 w550 w559 w562 w566 w569 w572 w575 w578 w583 w585 w589 w594 w601 w613 w625 w631 w646 w653 w663 w672 w676 w685 w700 w706 w707 w712] -> w70
      event Timeout {
        n41 = event-data() -> ()  [unwired: 1 in, 1 out]
      }
      event "scan_start": Value Change {
        n42 = event-data() -> ("NewVal"=w511:bool)  [unwired: 1 in]
        n43 = Select(t=T12."do3DScan", s=w511, f=enum16{"Standby", "doScan"}."Standby") -> (s? t:f=w513:T12)
      }
      event "live-scan": Value Change {
        n44 = event-data() -> ("NewVal"=w517:bool)  [unwired: 1 in]
        n45 = Select(t=T13."doLiveScan", s=w517, f=T13."Standby") -> (s? t:f=w518:T13)
      }
      event "counting_start": Value Change {
        n46 = event-data() -> ("NewVal"=w522:bool)  [unwired: 1 in]
        n47 = Select(t=T14."doCount", s=w522, f=T14."Standby") -> (s? t:f=w519:T14)
      }
      event "focus_start": Value Change {
        n48 = event-data() -> ("NewVal"=w525:bool)  [unwired: 1 in]
        n49 = Select(t=T15."doFocus", s=w525, f=T15."doFocus") -> (s? t:f=w526:T15)
      }
      event "pos-start_cursor": Value Change {
        n50 = event-data() -> ()  [unwired: 1 in, 1 out]
        n51 = property on="scan_image" class="IntGraph (strict)"() -> ("Cursor.Cursor X"=w532:dbl, "Cursor.Cursor Y"=w531:dbl)  [unwired: 2 in, 2 out]
        n52 = property on="pos-start_x" class="DigNum (strict)"("Value"=w532) -> ()  [unwired: 2 in, 2 out]
        n53 = property on="pos-start_y" class="DigNum (strict)"("Value"=w531) -> ()  [unwired: 2 in, 2 out]
      }
      event "pos-zero": Value Change {
        w535 = 0.0 ("pos-start_x")
        n54 = event-data() -> ()  [unwired: 1 in, 1 out]
        n55 = property on="pos-start_x" class="DigNum (strict)"("Value"=w535) -> ()  [unwired: 2 in, 2 out]
        n56 = property on="pos-start_y" class="DigNum (strict)"("Value"=w535) -> ()  [unwired: 2 in, 2 out]
      }
      event "cursor-reset": Value Change {
        n57 = event-data() -> ()  [unwired: 1 in, 1 out]
        n58 = property on="scan_image" class="IntGraph (strict)"() -> ("XScale.Maximum"=w548:dbl, "XScale.Minimum"=w543:dbl, "YScale.Maximum"=w539:dbl, "YScale.Minimum"=w538:dbl)  [unwired: 2 in, 2 out]
        n59 = Subtract(x=w548, y=w543) -> (x-y=w546:dbl)
        n60 = Subtract(x=w539, y=w538) -> (x-y=w542:dbl)
        n61 = Multiply(x=0.5 ("y"), y=w546) -> (x*y=w544:dbl)
        n62 = Multiply(x=0.5 ("y"), y=w542) -> (x*y=w540:dbl)
        n63 = Add(x=w544, y=w543) -> (x+y=w547:dbl)
        n64 = Add(x=w540, y=w538) -> (x+y=w537:dbl)
        n65 = property on="scan_image" class="IntGraph (strict)"("Cursor.Cursor X"=w547, "Cursor.Cursor Y"=w537) -> ()  [unwired: 2 in, 2 out]
      }
      event "objective": Value Change {
        n66 = event-data() -> ("NewVal"=w552:u16)  [unwired: 1 in]
        n67 = case shown="2" w552 {
          frame 0, Default {
            # "In this case, all distances\nare shown in volts."
            n68 = global read "GLOBAL_VAR.vi" "Kx_volt"() -> (w554:dbl)
            n69 = global read "GLOBAL_VAR.vi" "Ky_volt"() -> (w553:dbl)
            n70 = global write "GLOBAL_VAR.vi" "Kx"(w554) -> ()
            n71 = global write "GLOBAL_VAR.vi" "Ky"(w553) -> ()
          }
          frame 1 {
            # "100x"
            n72 = global read "GLOBAL_VAR.vi" "Kx_oil"() -> (w556:dbl)
            n73 = global read "GLOBAL_VAR.vi" "Ky_oil"() -> (w555:dbl)
            n74 = global write "GLOBAL_VAR.vi" "Kx"(w556) -> ()
            n75 = global write "GLOBAL_VAR.vi" "Ky"(w555) -> ()
          }
          frame 2 {
            n76 = global read "GLOBAL_VAR.vi" "Kx_air"() -> (w558:dbl)
            n77 = global read "GLOBAL_VAR.vi" "Ky_air"() -> (w557:dbl)
            n78 = global write "GLOBAL_VAR.vi" "Kx"(w558) -> ()
            n79 = global write "GLOBAL_VAR.vi" "Ky"(w557) -> ()
          }
        }
      }
      event "pos_z": Value Change {
        n80 = event-data() -> ("NewVal"=w560:dbl)  [unwired: 1 in]
        n81 = call "set_z.vi"("z_value_um"=w560) -> ()  [unwired: 10 in, 1 out]
        n82 = property on="focus_z" class="DigNum (strict)"("Value"=w560) -> ()  [unwired: 2 in, 2 out]
        n83 = property on="current_z" class="DigNum (strict)"("Value"=w560) -> ()  [unwired: 2 in, 2 out]
      }
      event "focus_z": Value Change {
        n84 = event-data() -> ("NewVal"=w563:dbl)  [unwired: 1 in]
        n85 = call "set_z.vi"("z_value_um"=w563) -> ()  [unwired: 10 in, 1 out]
        n86 = property on="pos_z" class="Slide (strict)"("Value"=w563) -> ()  [unwired: 2 in, 2 out]
        n87 = property on="current_z" class="DigNum (strict)"("Value"=w563) -> ()  [unwired: 2 in, 2 out]
      }
      event "focus_z_start", "focus_z_end": Value Change {
        n88 = event-data() -> ()  [unwired: 1 in, 1 out]
        n89 = property on="focus_z_end" class="DigNum (strict)"() -> ("Value"=w568:dbl)  [unwired: 2 in, 2 out]
        n90 = property on="focus_z_start" class="DigNum (strict)"() -> ("Value"=w567:dbl)  [unwired: 2 in, 2 out]
        n91 = property on="pos_z" class="Slide (strict)"("Scale.Maximum"=w568, "Scale.Minimum"=w567) -> ()  [unwired: 2 in, 2 out]
      }
      event "z-stack-set_from": Value Change {
        n92 = event-data() -> ()  [unwired: 1 in, 1 out]
        n93 = property on="current_z" class="DigNum (strict)"() -> ("Value"=w571:dbl)  [unwired: 2 in, 2 out]
        n94 = property on="z-stack_from" class="DigNum (strict)"("Value"=w571) -> ()  [unwired: 2 in, 2 out]
      }
      event "z-stack-set_to": Value Change {
        n95 = event-data() -> ()  [unwired: 1 in, 1 out]
        n96 = property on="current_z" class="DigNum (strict)"() -> ("Value"=w574:dbl)  [unwired: 2 in, 2 out]
        n97 = property on="z-stack_to" class="DigNum (strict)"("Value"=w574) -> ()  [unwired: 2 in, 2 out]
      }
      event "z-stack-set_center": Value Change {
        n98 = event-data() -> ()  [unwired: 1 in, 1 out]
        n99 = property on="current_z" class="DigNum (strict)"() -> ("Value"=w577:dbl)  [unwired: 2 in, 2 out]
        n100 = property on="z-stack_center" class="DigNum (strict)"("Value"=w577) -> ()  [unwired: 2 in, 2 out]
      }
      event "current_x", "current_y", "current_z": Value Change {
        n101 = event-data() -> ()  [unwired: 1 in, 1 out]
        n102 = call "set_xy.vi"("y_value_um"="current_y", "x_value_um"="current_x") -> ()  [unwired: 9 in, 1 out]
        n103 = call "set_z.vi"("z_value_um"="current_z") -> ()  [unwired: 10 in, 1 out]
      }
      event "z-stack_pos": Value Change {
        n104 = event-data() -> ()  [unwired: 1 in, 1 out]
      }
      event "z-stack_slices": Value Change {
        n105 = event-data() -> ("NewVal"=w588:i32)  [unwired: 1 in]
        n106 = property on="z-stack_pos" class="Slide (strict)"("Scale.Maximum"=w588, "Scale.Minimum"=1.0 ("Scale.Range:Minimum")) -> ()  [unwired: 2 in, 2 out]
      }
      event "esr_start": Value Change {
        n107 = event-data() -> ("NewVal"=w591:bool)  [unwired: 1 in]
        n108 = Select(t=T18."doESR", s=w591, f=T18."Standby") -> (s? t:f=w593:T18)
      }
      event "tile-scan_start": Value Change {
        n109 = event-data() -> ("NewVal"=w597:bool)  [unwired: 1 in]
        n110 = global read "GLOBAL_VAR.vi" "Motors-enable"() -> (w595:bool)
        n111 = And(x=w597, y=w595) -> (x .and. y?=w596:bool)
        n112 = Select(t=T19."doTileScan", s=w596, f=T19."Standby") -> (s? t:f=w600:T19)
      }
      event "timeseries-start": Value Change {
        n113 = event-data() -> ("NewVal"=w604:bool)  [unwired: 1 in]
        n114 = Select(t=T14."doTimeseries", s=w604, f=T14."Standby") -> (s? t:f=w605:T14)
      }
      event "upos-x", "upos-y": Value Change {
        n115 = event-data() -> ()  [unwired: 1 in, 1 out]
        n116 = property on="upos-x" class="DigNum (strict)"() -> ("Value"=w610:dbl)  [unwired: 2 in, 2 out]
        n117 = property on="upos-y" class="DigNum (strict)"() -> ("Value"=w609:dbl)  [unwired: 2 in, 2 out]
        n118 = property on="X Zero" class="DigNum (strict)"() -> ("Value"=w608:dbl)  [unwired: 2 in, 2 out]
        n119 = property on="Y Zero" class="DigNum (strict)"() -> ("Value"=w607:dbl)  [unwired: 2 in, 2 out]
        n120 = Subtract(x=w609, y=w607) -> (x-y=w612:dbl)
        n121 = Bundle(T20."domove", "Value"=w610, "Value"=w609, "Value"=0.0) -> (w615:T23)  [unwired: 1 in]
        n122 = Subtract(x=w610, y=w608) -> (x-y=w611:dbl)
        n123 = Enqueue Element(queue=w617, element=w615) -> (queue out=w613:refnum<queue>)  [unwired: 2 in, 2 out]
        n124 = property on="upos-xy_control" class="XYGraph (strict)"("Cursor.Cursor X"=w610, "Cursor.Cursor Y"=w609) -> ()  [unwired: 2 in, 2 out]
        n125 = property on="X Rel" class="DigNum (strict)"("Value"=w611) -> ()  [unwired: 2 in, 2 out]
        n126 = property on="Y Rel" class="DigNum (strict)"("Value"=w612) -> ()  [unwired: 2 in, 2 out]
      }
      event "X Rel", "Y Rel": Value Change {
        n127 = event-data() -> ()  [unwired: 1 in, 1 out]
        n128 = property on="X Rel" class="DigNum (strict)"() -> ("Value"=w624:dbl)  [unwired: 2 in, 2 out]
        n129 = property on="X Zero" class="DigNum (strict)"() -> ("Value"=w622:dbl)  [unwired: 2 in, 2 out]
        n130 = property on="Y Rel" class="DigNum (strict)"() -> ("Value"=w623:dbl)  [unwired: 2 in, 2 out]
        n131 = property on="Y Zero" class="DigNum (strict)"() -> ("Value"=w621:dbl)  [unwired: 2 in, 2 out]
        n132 = Add(x=w624, y=w622) -> (x+y=w620:dbl)
        n133 = Add(x=w623, y=w621) -> (x+y=w619:dbl)
        n134 = Bundle(T20."domove", w620, w619, "Value"=0.0) -> (w629:T24)  [unwired: 1 in]
        n135 = property on="upos-x" class="DigNum (strict)"("Value"=w620) -> ()  [unwired: 2 in, 2 out]
        n136 = property on="upos-y" class="DigNum (strict)"("Value"=w619) -> ()  [unwired: 2 in, 2 out]
        n137 = Enqueue Element(queue=w626, element=w629) -> (queue out=w625:refnum<queue>)  [unwired: 2 in, 2 out]
        n138 = property on="upos-xy_control" class="XYGraph (strict)"("Cursor.Cursor X"=w620, "Cursor.Cursor Y"=w619) -> ()  [unwired: 2 in, 2 out]
      }
      event "X Zero", "Y Zero": Value Change {
        n139 = event-data() -> ()  [unwired: 1 in, 1 out]
        n140 = property on="upos-x" class="DigNum (strict)"() -> ("Value"=w637:dbl)  [unwired: 2 in, 2 out]
        n141 = property on="X Zero" class="DigNum (strict)"() -> ("Value"=w633:dbl)  [unwired: 2 in, 2 out]
        n142 = property on="upos-y" class="DigNum (strict)"() -> ("Value"=w636:dbl)  [unwired: 2 in, 2 out]
        n143 = property on="Y Zero" class="DigNum (strict)"() -> ("Value"=w632:dbl)  [unwired: 2 in, 2 out]
        n144 = Subtract(x=w637, y=w633) -> (x-y=w635:dbl)
        n145 = Subtract(x=w636, y=w632) -> (x-y=w634:dbl)
        n146 = property on="X Rel" class="DigNum (strict)"("Value"=w635) -> ()  [unwired: 2 in, 2 out]
        n147 = property on="Y Rel" class="DigNum (strict)"("Value"=w634) -> ()  [unwired: 2 in, 2 out]
      }
      event "upos-xy_control": Cursor Move {
        n148 = event-data() -> ("CursLoc.X"=w644:dbl, "CursLoc.Y"=w643:dbl)  [unwired: 1 in]
        n149 = property on="X Zero" class="DigNum (strict)"() -> ("Value"=w640:dbl)  [unwired: 2 in, 2 out]
        n150 = property on="Y Zero" class="DigNum (strict)"() -> ("Value"=w639:dbl)  [unwired: 2 in, 2 out]
        n151 = property on="upos-x" class="DigNum (strict)"("Value"=w644) -> ()  [unwired: 2 in, 2 out]
        n152 = property on="upos-y" class="DigNum (strict)"("Value"=w643) -> ()  [unwired: 2 in, 2 out]
        n153 = Subtract(x=w644, y=w640) -> (x-y=w642:dbl)
        n154 = Subtract(x=w643, y=w639) -> (x-y=w641:dbl)
        n155 = Bundle(enum16{"standby", "domove", "dostop"}."standby", "X"=w644, "Y"=w643, 0.0) -> (w647:T25)  [unwired: 1 in]
        n156 = Enqueue Element(queue=w645, element=w647) -> (queue out=w646:refnum<queue>)  [unwired: 2 in, 2 out]
        n157 = property on="X Rel" class="DigNum (strict)"("Value"=w642) -> ()  [unwired: 2 in, 2 out]
        n158 = property on="Y Rel" class="DigNum (strict)"("Value"=w641) -> ()  [unwired: 2 in, 2 out]
      }
      event "upos-xy_control": Cursor Release {
        n159 = event-data() -> ()  [unwired: 1 in, 1 out]
        n160 = Bundle(enum16{"standby", "domove", "dostop", "exit"}."domove", "upos-x"="upos-x", "upos-y"="upos-y", 0.0) -> (w655:T26)  [unwired: 1 in]
        n161 = Enqueue Element(queue=w654, element=w655) -> (queue out=w653:refnum<queue>)  [unwired: 2 in, 2 out]
      }
      event "upos-stop": Value Change {
        n162 = event-data() -> ("NewVal"=w667:bool)  [unwired: 1 in]
        n163 = Select(t=enum16{"standby", "domove", "dostop", "exit"}."dostop", s=w667, f=enum16{"standby", "domove", "dostop", "exit"}."standby") -> (s? t:f=w661:enum16{"standby", "domove", "dostop", "exit"})
        n164 = Bundle(w661, 0.0, 0.0, 0.0) -> (w660:T27)  [unwired: 1 in]
        n165 = Enqueue Element(queue=w662, element=w660) -> (queue out=w663:refnum<queue>)  [unwired: 2 in, 2 out]
      }
      event User Event {
        n166 = event-data() -> ("status_x"=→"upos-state_x":dbl, "status_y"=→"upos-state_y":dbl, "pos_x"=w670:dbl, "pos_y"=w669:dbl)  [unwired: 1 in, 2 out]
        "upos-cpos_y" <- w669
        "upos-cpos_x" <- w670
        n167 = Bundle("pos_x"=w670, "pos_y"=w669) -> (w668:cluster{"pos_x":dbl, "pos_y":dbl})  [unwired: 1 in]
        n168 = Build Array(w668) -> (w671:cluster{"pos_x":dbl, "pos_y":dbl}[])
        n169 = property on="upos-xy_control" class="XYGraph (strict)"("Value"=w671) -> ()  [unwired: 2 in, 2 out]
      }
      event "stop": Value Change {
        n170 = event-data() -> ("NewVal"=w675:bool)  [unwired: 1 in]
        n171 = Select(t=enum16{"standby", "domove", "dostop", "exit"}."exit", s=w675, f=enum16{"standby", "domove", "dostop", "exit"}."standby") -> (s? t:f=w681:enum16{"standby", "domove", "dostop", "exit"})
        n172 = Bundle(w681, 0.0, 0.0, 0.0) -> (w680:T27)  [unwired: 1 in]
        n173 = Enqueue Element(queue=w677, element=w680) -> (queue out=w676:refnum<queue>)  [unwired: 2 in, 2 out]
      }
      event "timeseries-stopdate", "timeseries-period": Value Change {
        n174 = event-data() -> ()  [unwired: 1 in, 1 out]
        n175 = property on="timeseries-stopdate" class="AbsTime (strict)"() -> ("Value"=w692:timestamp)  [unwired: 2 in, 2 out]
        n176 = Get Date/Time In Seconds() -> (seconds since 1Jan1904=w691:timestamp)
        n177 = Subtract(x=w692, y=w691) -> (x-y=w690:dbl)
        n178 = Greater Than 0?(x=w690) -> (x > 0?=w689:bool)
        n179 = case shown="True" w689 {
          tunnel: w690 -> [_ w698]
          tunnel: [0.0 w696] -> w688
          tunnel: ["00:00:00" ("HH:MM:SS") w695] -> w687
          frame False {
          }
          frame True {
            n180 = property on="timeseries-period" class="DigNum (strict)"() -> ("Value"=w699:dbl)  [unwired: 2 in, 2 out]
            n181 = Divide(x=w698, y=w699) -> (x/y=w697:dbl)
            n182 = call "seconds2time.vi"("seconds"=w698) -> ("HH:MM:SS"=w695:string)  [unwired: 10 in]
            n183 = Round To Nearest(number=w697) -> (nearest integer value=w696:dbl)
          }
        }
        "timeseries-total_images" <- w688
        "timeseries-rem_time" <- w687
        "timeseries-current_image" <- 0.0 ("timeseries-current_image")
      }
      event "laser_on-off": Value Change {
        n184 = event-data() -> ("NewVal"=w701:bool)  [unwired: 1 in]
        n185 = call "laserON-OFF.vi"("ON-OFF"=w701) -> ()  [unwired: 10 in, 1 out]
      }
      event "T1_open": Value Change {
        n186 = event-data() -> ("NewVal"=w705:bool)  [unwired: 1 in]
        n187 = Select(t=T21."doT1", s=w705, f=T21."Standby") -> (s? t:f=w704:T21)
      }
      event "file_save": Value Change {
        n188 = event-data() -> ("NewVal"=w708:bool)  [unwired: 1 in]
        n189 = Select(t=T22."saveImage", s=w708, f=T22."Standby") -> (s? t:f=w711:T22)
      }
      event "recenter": Value Change {
        n190 = event-data() -> ("NewVal"=w716:bool)  [unwired: 1 in]
        n191 = Select(t=T16."doRecenter", s=w716, f=T16."Standby") -> (s? t:f=w713:T16)
      }
    }
    n192 = control-ref of="scan_image"() -> (w79:refnum<vi>)
    n193 = control-ref of="scan_start"() -> (w78:refnum<vi>)
    n194 = control-ref of="pos-start_y"() -> (w77:refnum<vi>)
    n195 = control-ref of="pos-start_x"() -> (w76:refnum<vi>)
    n196 = case shown="\"doRecenter\"" w86 {
      tunnel: w78 -> [_ _ _ _ w264 _ _ _ _ _ _ _]
      tunnel: w77 -> [_ _ _ _ _ _ _ _ _ _ _ _]
      tunnel: w76 -> [_ _ _ _ _ _ _ _ _ _ _ _]
      tunnel: [w131 w174 w195 w216 w237 w303 w334 w379 w424 w464 w476 w492] -> w85
      tunnel: w84 -> [w131 w174 w195 w216 _ w303 w334 w379 w424 w464 w476 w492]
      tunnel: "pixel_dwell_ms" -> [w130 _ _ _ w232 _ _ w361 w418 w461 _ _]
      tunnel: "scan_direction" -> [_ _ _ _ w249 _ _ w360 w411 _ _ _]
      tunnel: "frame_size_x_px" -> [w129 _ _ _ w233 _ _ w359 w413 _ _ _]
      tunnel: "pos_start" -> [_ _ _ w213 w248 _ _ w358 w412 _ _ _]
      tunnel: w79 -> [_ _ _ w215 w235 _ _ w357 w400 w455 _ _]
      tunnel: "image_size_x_um" -> [w128 _ _ w214 w234 _ _ w343 w414 w462 _ _]
      tunnel: w71 -> [_ _ _ _ _ _ _ w355 _ _ _ _]
      tunnel: w70 -> [_ _ _ _ _ _ _ w354 _ _ _ _]
      tunnel: "focus_z_start" -> [_ _ w194 _ _ _ _ w352 _ _ _ _]
      tunnel: "focus_z_end" -> [_ _ w193 _ _ _ _ w351 _ _ _ _]
      tunnel: "focus_q_steps" -> [_ _ w192 _ _ _ _ w350 _ _ _ _]
      tunnel: "focus_dwell_ms" -> [_ _ w191 _ _ _ _ w349 _ _ _ _]
      tunnel: "XY Max focus?" -> [_ _ _ _ _ _ _ w347 _ _ _ _]
      tunnel: "focus_z" -> [_ _ _ _ w240 _ w324 _ w404 w434 w471 _]
      tunnel: w62 -> [w96 w168 w190 w212 w245 w299 w306 w340 w391 w470 w478 w491]
      tunnel: w61 -> [w95 w167 w189 w211 w244 w298 w305 w339 w390 w469 w477 w490]
      tunnel: [w94 w168 w190 w212 w245 w299 w306 w340 w391 w470 w478 w491] -> w60
      tunnel: [w93 w167 w189 w211 w244 w298 w305 w339 w390 w469 w477 w490] -> w59
      tunnel: "file_path" -> [_ _ _ _ w243 _ _ _ _ w466 _ _]
      tunnel: "file_name" -> [_ _ _ _ w242 _ _ _ _ w465 _ _]
      tunnel: "X Zero" -> [_ _ _ _ _ _ _ _ _ w447 _ _]
      tunnel: "Y Zero" -> [_ _ _ _ _ _ _ _ _ w446 _ _]
      tunnel: "pos-start_x" -> [_ _ _ _ w231 _ _ w337 _ w444 _ _]
      tunnel: "pos-start_y" -> [_ _ _ _ w230 _ _ w336 _ w443 _ _]
      tunnel: [w87 w166 w188 w210 w238 w297 w304 w335 w389 w435 w479 w489] -> w52
      tunnel: w51 -> [_ w166 w188 w210 w238 w297 w304 w335 w389 w435 w479 w489]
      tunnel: "objective" -> [_ _ _ _ w241 _ _ _ _ _ _ _]
      tunnel: "file_autosave" -> [_ _ _ _ w236 _ _ _ _ _ _ _]
      frame "Standby", Default {
        w108 = 1000.0 ("y")
        # "Power in the sample"
        # "Updates the remaining time when time series are running"
        # "Calculation of the distance between slices in a z-stack"
        # "This section shows the x-section and y-section views of the image in the the graphs"
        # "This section calculates the pixel size and the total time per image."
        n197 = property on="scan_image" class="IntGraph (strict)"() -> ("Value"=w145:dbl[][], "Cursor.Cursor X"=w138:dbl, "XScale.Offset"=w107:dbl, "XScale.Multiplier"=w127:dbl, "Cursor.Cursor Y"=w137:dbl, "YScale.Offset"=w106:dbl, "YScale.Multiplier"=w119:dbl, "Cursor.Cursor X"=w102:dbl, "Cursor.Cursor Y"=w103:dbl)  [unwired: 2 in, 2 out]
        n198 = property on="X Rel" class="DigNum (strict)"() -> ("Value"=w109:dbl)  [unwired: 2 in, 2 out]
        n199 = property on="Y Rel" class="DigNum (strict)"() -> ("Value"=w110:dbl)  [unwired: 2 in, 2 out]
        n200 = Multiply(x=w109, y=w108) -> (x*y=w100:dbl)
        n201 = Multiply(x=w110, y=w108) -> (x*y=w98:dbl)
        n202 = Square(x=w129) -> (x^2=w153:i32)
        n203 = Divide(x=w128, y=w129) -> (x/y=→"pixel_size_x_um":dbl)
        n204 = Divide(x=w128, y=w129) -> (x/y=→"pixel_size_y_um":dbl)
        n205 = Multiply(x=w153, y=w130) -> (x*y=w148:dbl)
        n206 = Add(x=w107, y=w98) -> (x+y=w105:dbl)
        n207 = Subtract(x=w138, y=w107) -> (x-y=w147:dbl)
        n208 = Subtract(x=w137, y=w106) -> (x-y=w144:dbl)
        n209 = Add(x=w106, y=w100) -> (x+y=w104:dbl)
        n210 = Add(x=w102, y=w100) -> (x+y=→"X":dbl)
        n211 = Add(x=w103, y=w98) -> (x+y=→"Y":dbl)
        n212 = Divide(x=w148, y=1000.0) -> (x/y=→"time_frame_s":dbl)
        n213 = Divide(x=w147, y=w127) -> (x/y=w146:dbl)
        n214 = Divide(x=w144, y=w119) -> (x/y=w143:dbl)
        n215 = Round To Nearest(number=w146) -> (nearest integer value=w124:dbl)
        n216 = Round To Nearest(number=w143) -> (nearest integer value=w142:dbl)
        n217 = property on="timeseries-start" class="Bool (strict)"() -> ("Value"=w97:bool)  [unwired: 2 in, 2 out]
        n218 = Index Array(array=w145, index (row)=w124) -> (element=w117:dbl[])  [unwired: 1 in]
        n219 = Index Array(array=w145, index (col)=w142) -> (element=w120:dbl[])  [unwired: 1 in]
        n220 = global read "GLOBAL_VAR.vi" "power_factor"() -> (w88:dbl)
        n221 = case shown="False" w97 {
          frame False {
          }
          frame True {
            n222 = property on="timeseries-stopdate" class="AbsTime (strict)"() -> ("Value"=w158:timestamp)  [unwired: 2 in, 2 out]
            n223 = Get Date/Time In Seconds() -> (seconds since 1Jan1904=w157:timestamp)
            n224 = Subtract(x=w158, y=w157) -> (x-y=w155:dbl)
            n225 = Greater Than 0?(x=w155) -> (x > 0?=w156:bool)
            n226 = case shown="True" w156 {
              tunnel: w155 -> [_ w161]
              tunnel: ["00:00:00" ("HH:MM:SS") w160] -> w154
              frame False {
              }
              frame True {
                n227 = call "seconds2time.vi"("seconds"=w161) -> ("HH:MM:SS"=w160:string)  [unwired: 10 in]
              }
            }
            n228 = property on="timeseries-rem_time" class="Str"("Value"=w154) -> ()  [unwired: 2 in, 2 out]
          }
        }
        n229 = property on="Z-stack_tabs" class="TabCtl (strict)"() -> ("Value"=w139:enum32{"From-To", "Centering"})  [unwired: 2 in, 2 out]
        n230 = Array Size(array=w117) -> (size(s)=w125:i32)
        n231 = Array Size(array=w120) -> (size(s)=w122:i32)
        n232 = call <instrlib>:"PM100D Measure Power.vi"("error in (no error)"=w95, "instrument handle"=w96) -> ("error out"=w93:errorcluster, "Power"=w92:dbl, "instrument handle out"=w94:refnum<visa-resource-name>)  [unwired: 7 in]
        n233 = Decrement(x=w125) -> (x-1=w112:i32)
        n234 = Decrement(x=w122) -> (x-1=w111:i32)
        n235 = case shown="\"From-To\", Default" w139 {
          tunnel: [w162 w165] -> w140
          frame "From-To", Default {
            n236 = property on="z-stack_to" class="DigNum (strict)"() -> ("Value"=w164:dbl)  [unwired: 2 in, 2 out]
            n237 = property on="z-stack_from" class="DigNum (strict)"() -> ("Value"=w163:dbl)  [unwired: 2 in, 2 out]
            n238 = Subtract(x=w164, y=w163) -> (x-y=w162:dbl)
          }
          frame "Centering" {
            n239 = property on="z-stack_size" class="DigNum (strict)"() -> ("Value"=w165:dbl)  [unwired: 2 in, 2 out]
          }
        }
        n240 = Multiply(x=w112, y=w127) -> (x*y=w126:dbl)
        n241 = Multiply(x=w111, y=w119) -> (x*y=w123:dbl)
        n242 = Multiply(x=w92, y=w88) -> (x*y=w91:dbl)
        n243 = Add(x=w126, y=w105) -> (x+y=w114:dbl)
        n244 = Add(x=w123, y=w104) -> (x+y=w113:dbl)
        n245 = property on="z-stack_slices" class="DigNum (strict)"() -> ("Value"=w141:i32)  [unwired: 2 in, 2 out]
        n246 = In Range and Coerce(upper limit=inf, x=w91, lower limit=0.0) -> (coerced(x)=w87:dbl)  [unwired: 1 out]
        "Laser power [mW]" <- w87
        n247 = call-poly <vilib>:"Ramp Pattern.vi"("start"=w105, "end"=w114, "samples"=w125) -> ("Ramp Pattern"=w118:dbl[])  [unwired: 7 in, 1 out]
        n248 = call-poly <vilib>:"Ramp Pattern.vi"("start"=w104, "end"=w113, "samples"=w122) -> ("Ramp Pattern"=w121:dbl[])  [unwired: 7 in, 1 out]
        n249 = Decrement(x=w141) -> (x-1=w132:i32)
        n250 = Bundle("Value"=w117, "Ramp Pattern"=w118) -> (→"XY Graph":cluster{"Value":dbl[], "Ramp Pattern":dbl[]})  [unwired: 1 in]
        n251 = Bundle("Ramp Pattern"=w121, "Value"=w120) -> (→"XY Graph 2":cluster{"Ramp Pattern":dbl[], "Value":dbl[]})  [unwired: 1 in]
        n252 = Divide(x=w140, y=w132) -> (x/y=w136:dbl)
        n253 = Greater Than 0?(x=w132) -> (x > 0?=w133:bool)
        n254 = property on="XY Graph" class="XYGraph (strict)"("YScale.Maximum"=w114, "YScale.Minimum"=w105) -> ()  [unwired: 2 in, 2 out]
        n255 = property on="XY Graph 2" class="XYGraph (strict)"("XScale.Maximum"=w113, "XScale.Minimum"=w104) -> ()  [unwired: 2 in, 2 out]
        n256 = Select(t=w136, s=w133, f=0.0) -> (s? t:f=→"z-stack_step_size":dbl)
        "frame_size_y_px" <- w129
        "image_size_y_um" <- w128
      }
      frame "doCount" {
        n257 = control-ref of="wavechart_01"() -> (w175:refnum<vi>)
        n258 = control-ref of="counts"() -> (w176:refnum<vi>)
        n259 = control-ref of="scan_image"() -> (w177:refnum<vi>)
        n260 = Open VI Reference(type specifier VI Refnum (for type only)=refnum<vi> refnum, vi path=path "src/doCount.vi", options=128) -> (vi reference=w182:refnum<vi>, error out=w183:errorcluster)  [unwired: 3 in]
        n261 = control-ref of="counting_start"() -> (w178:refnum<vi>)
        n262 = Multiply(x="counts_dwell_time", y=0.001) -> (x*y=w173:dbl)
        n263 = call-by-ref "Start Asynchronous Call"(reference=w182, error in=w183, "counts_out_ref_chart"=w175, "counts_out_ref"=w176, "enable"=w178, "Acquisition time [s]"=w173, "cursors_ref"=w177) -> (reference out=w184:refnum<vi>, error out=w185:errorcluster)  [unwired: 7 in]
        n264 = property on="wavechart_01" class="WFChart (strict)"("XScale.Multiplier"=1.0 ("X Scale.Offset and Multiplier:Multiplier"), "XScale.Offset"=0.0 ("X Scale.Offset and Multiplier:Offset"), "History Data"=dbl[] []) -> ()  [unwired: 2 in, 2 out]
        n265 = Close Reference(reference=w184, error in (no error)=w185) -> ()  [unwired: 1 out]
      }
      frame "doFocus" {
        n266 = property on="scan_image" class="IntGraph (strict)"() -> ("Cursor.Cursor X"=w198:dbl, "Cursor.Cursor Y"=w197:dbl)  [unwired: 2 in, 2 out]
        n267 = Decrement(x=w192) -> (x-1=w200:i32)
        n268 = Subtract(x=w193, y=w194) -> (x-y=w201:dbl)
        n269 = call "set_xy.vi"("y_value_um"=w197, "x_value_um"=w198) -> ("error out"=w187:errorcluster)  [unwired: 9 in]
        n270 = control-ref of="wavechart_01"() -> (w203:refnum<vi>)
        n271 = Divide(x=w201, y=w200) -> (x/y=w199:dbl)
        n272 = flat-sequence {
          tunnel: w203 -> [w209]
          tunnel: [w208] -> w196
          tunnel: w194 -> [w207]
          tunnel: w193 -> [w206]
          tunnel: w192 -> [w205]
          tunnel: w191 -> [w204]
          tunnel: w187 -> [_]
          frame #0 {
            n273 = call "auto_focus.vi"("counts"=w209, "dwell_time_ms"=w204, "q_steps"=w205, "z_end"=w206, "z_start"=w207) -> ("z_focus"=w208:dbl)  [unwired: 5 in, 1 out]
          }
        }
        n274 = property on="wavechart_01" class="WFChart (strict)"("History Data"=dbl[] [], "XScale.Offset"=w194, "XScale.Multiplier"=w199) -> ()  [unwired: 2 in, 2 out]
        n275 = property on="focus_z" class="DigNum (strict)"("Val(Sgnl)"=w196) -> ()  [unwired: 2 in, 2 out]
        n276 = property on="current_z" class="DigNum (strict)"("Value"=w196) -> ()  [unwired: 2 in, 2 out]
      }
      frame "doLiveScan" {
        n277 = Open VI Reference(type specifier VI Refnum (for type only)=refnum<vi> refnum, vi path=path "src/live_scanner.vi", options=128) -> (vi reference=w224:refnum<vi>, error out=w228:errorcluster)  [unwired: 3 in]
        n278 = control-ref of="live-scan"() -> (w221:refnum<vi>)
        n279 = control-ref of="pos-start_y"() -> (w222:refnum<vi>)
        n280 = control-ref of="pos-start_x"() -> (w223:refnum<vi>)
        n281 = call-by-ref "Start Asynchronous Call"(reference=w224, error in=w228, "live_pixel_dwell_ms"="live_pixel_dwell_ms", "pos-start_x"=w223, "pos-start_y"=w222, "enable"=w221, "live_frame_size_x_px"="live_frame_size_x_px", "image_size_x_um"=w214, "pos_start"=w213, "live_scan_direction"="live_scan_direction", "IntensityGraph in"=w215) -> (reference out=w227:refnum<vi>, error out=w226:errorcluster)  [unwired: 6 in, 1 out]
        n282 = Close Reference(reference=w227, error in (no error)=w226) -> ()  [unwired: 1 out]
      }
      frame "do3DScan" {
        n283 = Bundle("pos-start_x"=w231, "pos-start_y"=w230, "focus_z"=w240) -> (w239:T28)  [unwired: 1 in]
        n284 = case shown="\"Centering\"" "Z-stack_tabs" {
          tunnel: ["z-stack_from" w293] -> w260
          tunnel: ["z-stack_to" w294] -> w259
          frame "From-To", Default {
          }
          frame "Centering" {
            n285 = Multiply(x="z-stack_size", y=0.5) -> (x*y=w291:dbl)
            n286 = Subtract(x="z-stack_center", y=w291) -> (x-y=w293:dbl)
            n287 = Add(x="z-stack_center", y=w291) -> (x+y=w294:dbl)
          }
        }
        n288 = Open VI Reference(type specifier VI Refnum (for type only)=refnum<vi> refnum, vi path=path "src/3D_scanner.vi", options=256) -> (vi reference=w257:refnum<vi>, error out=w254:errorcluster)  [unwired: 3 in]
        n289 = call-by-ref "Start Asynchronous Call"(reference=w257, error in=w254, "pixel_dwell_ms"=w232, "pos-start_x"=w231, "pos-start_y"=w230, "enable"=w264, "frame_size_x_px"=w233, "image_size_x_um"=w234, "pos_start"=w248, "z-stack_enable"="Z-stack_enable", "scan_direction"=w249, "IntensityGraph in"=w235, "z_start"=w260, "z_end"=w259, "z_q_slices"="z-stack_slices") -> ()  [unwired: 2 in, 3 out]
        n290 = call-by-ref "Wait On Asynchronous Call"(reference=w257, error in=w254) -> (reference out=w256:refnum<vi>, error out=w255:errorcluster, "image_out"=w237:dbl[][][])  [unwired: 15 in]
        n291 = case shown="True" w236 {
          tunnel: w243 -> [_ w286]
          tunnel: w242 -> [_ w285]
          tunnel: w234 -> [_ w284]
          tunnel: w232 -> [_ w282]
          tunnel: w241 -> [_ w278]
          tunnel: w239 -> [_ w275]
          tunnel: w238 -> [_ w274]
          tunnel: w237 -> [_ w273]
          frame False {
          }
          frame True {
            w288 = T29 {"file_path"=path "", "file_name"="", "image"=[], "image_size_xy"={"image_size_x_um"=1.0, "image_size_y_um"=1.0}, "pixel_dwell_time_ms"=1.0, "Laser_power_mW"=1.0, "pixel_size"=0.0, "tile_ij"={"tile_i"=0, "tile_j"=0}, "Objective"="", "ColorMarkers"=[], "timestamp"=timestamp(0 s since 1904-01-01), "micro-position-xyz"={"micro-position_x_mm"=1.0, "micro-position_y_mm"=1.0, "micro-position_z_mm"=1.0}, "zero_xyz"={"zero_x_mm"=0.0, "zero_y_mm"=0.0, "zero_z_mm"=0.0}, "nano-position-xyz"={"nano-position_x_V"=1.0, "nano-position_y_V"=1.0, "nano-position_z_V"=1.0}, "Kxyz"={"Kx_V/um"=1.0, "Ky_V/um"=1.0, "Kz_V/um"=1.0}}  # image_info
            n292 = property on="scan_image" class="IntGraph (strict)"() -> ("ZScale.MarkerVals[]"=w277:cluster{dbl, u32}[])  [unwired: 2 in, 2 out]
            n293 = property on="objective" class="Ring (strict)"() -> ("Strings []"=w280:string[])  [unwired: 2 in, 2 out]
            n294 = global read "GLOBAL_VAR.vi" "Ky"() -> (w271:dbl)
            n295 = global read "GLOBAL_VAR.vi" "Kx"() -> (w270:dbl)
            n296 = global read "GLOBAL_VAR.vi" "Kz"() -> (w272:dbl)
            n297 = property on="pixel_size_x_um" class="DigNum (strict)"() -> ("Value"=w281:dbl)  [unwired: 2 in, 2 out]
            n298 = Bundle("image_size_x_um"=w284, "image_size_x_um"=w284) -> (w283:T30)  [unwired: 1 in]
            n299 = Index Array(array=w280, index=w278) -> (element=w279:string)
            n300 = Get Date/Time In Seconds() -> (seconds since 1Jan1904=w276:timestamp)
            n301 = Bundle("Kx"=w270, "Ky"=w271, "Kz"=w272) -> (w269:cluster{"Kx":dbl, "Ky":dbl, "Kz":dbl})  [unwired: 1 in]
            n302 = Bundle By Name(cluster=w288, "image"=w273, "nano-position-xyz"=w275, "file_path"=w286, "file_name"=w285, "image_size_xy"=w283, "pixel_dwell_time_ms"=w282, "pixel_size"=w281, "Objective"=w279, "ColorMarkers"=w277, "timestamp"=w276, "Kxyz"=w269, "Laser_power_mW"=w274) -> (w287:T29)
            n303 = call "saveImage.vi"("save_txt"=TRUE ("save_tiff"), "save_tiff"=TRUE, "image_info"=w287) -> ()  [unwired: 9 in]
          }
        }
        n304 = Array Size(array=w237) -> (size(s)=w253:i32[])
        n305 = Close Reference(reference=w256, error in (no error)=w255) -> ()  [unwired: 1 out]
        n306 = Index Array(array=w253, index=0) -> (element=w251:i32)
        n307 = property on="z-stack_pos" class="Slide (strict)"("Scale.Maximum"=w251, "Scale.Minimum"=1.0 ("Scale.Range:Minimum")) -> (error out=w247:errorcluster)  [unwired: 2 in, 1 out]
        n308 = property on="scan_start" class="Bool (strict)"(error in=w247, "Value"=FALSE ("scan_start")) -> ()  [unwired: 1 in, 2 out]
      }
      frame "changeZslice" {
        n309 = Decrement(x="z-stack_pos") -> (x-1=w301:i32)
        n310 = Index Array(array=w303, index (dim 0)=w301) -> (element=→"scan_image":dbl[][])  [unwired: 2 in]
      }
      frame "doESR" {
        n311 = property on="scan_image" class="IntGraph (strict)"() -> ("Cursor.Cursor X"=w326:dbl, "Cursor.Cursor Y"=w325:dbl)  [unwired: 2 in, 2 out]
        n312 = Open VI Reference(type specifier VI Refnum (for type only)=refnum<vi> refnum, vi path=path "src/ESR/doESR.vi", options=128) -> (vi reference=w331:refnum<vi>, error out=w330:errorcluster)  [unwired: 3 in]
        n313 = Bundle("esr_repetitions"="esr_repetitions", "esr_power"="esr_power", "esr_freq_start"="esr_freq_start", "esr_freq_stop"="esr_freq_stop", "esr_step_size"="esr_step_size", "esr_dwell_time"="esr_dwell_time") -> (w308:T31)  [unwired: 1 in]
        n314 = Bundle("Cursor.Cursor X"=w326, "Cursor.Cursor Y"=w325, "focus_z"=w324) -> (w323:T32)  [unwired: 1 in]
        n315 = Subtract(x="esr_freq_stop", y="esr_freq_start") -> (x-y=w317:ext)
        n316 = Divide(x=w317, y="esr_step_size") -> (x/y=w316:ext)
        n317 = Compound Arithmetic op=MULTIPLY("esr_repetitions", w316, "esr_dwell_time") -> (→"esr_total_time":ext)
        n318 = control-ref of="esr_current_run"() -> (w322:refnum<vi>)
        n319 = control-ref of="ESR_stack"() -> (w307:refnum<vi>)
        n320 = call-by-ref "Start Asynchronous Call"(reference=w331, error in=w330, "IntGraph Refnum"=w307, "current_run_ref"=w322, "generator_enable"="esr_out_enable", "sweep_parameters"=w308, "position_xyz"=w323) -> (reference out=w327:refnum<vi>, error out=w328:errorcluster)  [unwired: 7 in]
        n321 = property on="esr_repetitions" class="DigNum (strict)"() -> ("Value"=w318:i32)  [unwired: 2 in, 2 out]
        n322 = property on="esr_current_run" class="DigNum (strict)"() -> ("Value"=w319:i32)  [unwired: 2 in, 2 out]
        n323 = Close Reference(reference=w327, error in (no error)=w328) -> ()  [unwired: 1 out]
        n324 = Subtract(x=w318, y=w319) -> (x-y=→"esr_remain":i32)
        "esr_power_led" <- "esr_out_enable"
      }
      frame "doTileScan" {
        n325 = Bundle("pos-start_x"=w337, "pos-start_y"=w336) -> (w338:cluster{"pos-start_x":dbl, "pos-start_y":dbl})  [unwired: 1 in]
        n326 = Bundle By Name(cluster=T9 {"z_start"=0.0, "z_end"=0.0, "q_steps"=0, "dwell_time_ms"=0.0} ("Focus (Piezo)"), "z_start"=w352, "z_end"=w351, "q_steps"=w350, "dwell_time_ms"=w349) -> (w348:T9)
        n327 = Bundle("tile_start_x_mm"="tile_start_x_mm", "tile_start_y_mm"="tile_start_y_mm") -> (w376:T33)  [unwired: 1 in]
        n328 = Multiply(x=w376, y=1000.0 ("tile_start_y_mm")) -> (x*y=w366:T33)
        n329 = case shown="\"tiles\", Default" "tile_tiles-size" {
          tunnel: w366 -> [w383 w388]
          tunnel: [w384 w387] -> w365
          tunnel: w343 -> [w382 _]
          frame "tiles", Default {
            n330 = Decrement(x="tile_q-tiles_x") -> (x-1=w381:dbl)
            n331 = Multiply(x=w382, y=w381) -> (x*y=w385:dbl)
            n332 = Add(x=w383, y=w385) -> (x+y=w384:T33)
            "tile_q-tiles_y" <- "tile_q-tiles_x"
          }
          frame "size" {
            n333 = Add(x=w388, y="tile_size_x_um") -> (x+y=w387:T33)
            "tile_size_y_um" <- "tile_size_x_um"
          }
        }
        n334 = Bundle By Name(cluster=T10 {"image_size"=0.0, "image_xy_start"={"image-x_start"=0.0, "image-y_start"=0.0}, "pixel_dwell_ms"=0.0, "frame_size_x_px"=0, "scan_direction"=enum."0", "pos_start"=enum."bottom-left"} ("Image (mirrors)"), "image_size"=w343, "image_xy_start"=w338, "pixel_dwell_ms"=w361, "frame_size_x_px"=w359, "scan_direction"=w360, "pos_start"=w358) -> (w362:T10)
        n335 = property on="X Zero" class="DigNum (strict)"() -> ("Value"=w345:dbl)  [unwired: 2 in, 2 out]
        n336 = property on="Y Zero" class="DigNum (strict)"() -> ("Value"=w344:dbl)  [unwired: 2 in, 2 out]
        n337 = Open VI Reference(type specifier VI Refnum (for type only)=refnum<vi> refnum, vi path=path "src/doTileScan.vi", options=128) -> (vi reference=w372:refnum<vi>, error out=w369:errorcluster)  [unwired: 3 in]
        n338 = Bundle("Value"=w345, "Value"=w344) -> (w342:cluster{"Value":dbl, "Value":dbl})  [unwired: 1 in]
        n339 = Bundle By Name(cluster=T8 {"overlap"=0.0, "pos-xy_start"={"pos-x_start"=0.0, "pos-y_start"=0.0}, "pos-xy_end"={"pos-x_end"=0.0, "pos-y_end"=0.0}, "pos-xy_ref"={"pos-x_start"=0.0, "pos-y_start"=0.0}} ("Positioners (motors)"), "overlap"="tiles-overlap", "pos-xy_start"=w366, "pos-xy_end"=w365, "pos-xy_ref"=w342) -> (w341:T8)
        n340 = control-ref of="wavechart_01"() -> (w356:refnum<vi>)
        n341 = call-by-ref "Start Asynchronous Call"(reference=w372, error in=w369, "Positioners (motors)"=w341, "IntensityGraph in"=w357, "status-event"=w355, "Image (mirrors)"=w362, "Focus (Piezo)"=w348, "XY Max?"=w347, "queue-commands"=w354, "WFChart Refnum"=w356) -> (reference out=w368:refnum<vi>, error out=w367:errorcluster)  [unwired: 8 in]
        n342 = Close Reference(reference=w368, error in (no error)=w367) -> ()  [unwired: 1 out]
      }
      frame "doTimeseries" {
        n343 = property on="Z-stack_tabs" class="TabCtl (strict)"() -> ("Value"=w410:enum32{"From-To", "Centering"})  [unwired: 2 in, 2 out]
        n344 = property on="pos-start_x" class="DigNum (strict)"() -> ("Value"=w423:dbl)  [unwired: 2 in, 2 out]
        n345 = property on="pos-start_y" class="DigNum (strict)"() -> ("Value"=w422:dbl)  [unwired: 2 in, 2 out]
        n346 = case shown="\"Centering\"" w410 {
          tunnel: [w427 w429] -> w409
          tunnel: [w426 w428] -> w408
          frame "From-To", Default {
            n347 = property on="z-stack_from" class="DigNum (strict)"() -> ("Value"=w427:dbl)  [unwired: 2 in, 2 out]
            n348 = property on="z-stack_to" class="DigNum (strict)"() -> ("Value"=w426:dbl)  [unwired: 2 in, 2 out]
          }
          frame "Centering" {
            n349 = property on="z-stack_center" class="DigNum (strict)"() -> ("Value"=w433:dbl)  [unwired: 2 in, 2 out]
            n350 = property on="z-stack_size" class="DigNum (strict)"() -> ("Value"=w432:dbl)  [unwired: 2 in, 2 out]
            n351 = Multiply(x=w432, y=0.5) -> (x*y=w431:dbl)
            n352 = Subtract(x=w433, y=w431) -> (x-y=w429:dbl)
            n353 = Add(x=w433, y=w431) -> (x+y=w428:dbl)
          }
        }
        n354 = Bundle("Value"=w423, "Value"=w422, "focus_z"=w404) -> (w415:cluster{"Value":dbl, "Value":dbl, "focus_z":dbl})  [unwired: 1 in]
        n355 = Open VI Reference(type specifier VI Refnum (for type only)=refnum<vi> refnum, vi path=path "src/doTimeSeries-3D.vi", options=256) -> (vi reference=w395:refnum<vi>, error out=w396:errorcluster)  [unwired: 3 in]
        n356 = property on="z-stack_slices" class="DigNum (strict)"() -> ("Value"=w407:i32)  [unwired: 2 in, 2 out]
        n357 = property on="Z-stack_enable" class="Bool (strict)"() -> ("Value"=w406:bool)  [unwired: 2 in, 2 out]
        n358 = call-by-ref "Wait On Asynchronous Call"(reference=w395, error in=w396) -> (reference out=w394:refnum<vi>, error out=w393:errorcluster, "return"=w392:enum16{"Error", "OK"})  [unwired: 15 in]
        n359 = Bundle("Value"=w409, "Value"=w408, "Value"=w407, "Value"=w406) -> (w405:T34)  [unwired: 1 in]
        n360 = control-ref of="timeseries-current_image"() -> (w398:refnum<vi>)
        n361 = control-ref of="timeseries-start"() -> (w401:refnum<vi>)
        n362 = control-ref of="timeseries-next_scan"() -> (w399:refnum<vi>)
        n363 = control-ref of="timeseries-rem_time"() -> (w397:refnum<vi>)
        n364 = Close Reference(reference=w394, error in (no error)=w393) -> ()  [unwired: 1 out]
        n365 = flat-sequence {
          tunnel: w392 -> [_]
          frame #0 {
            n366 = property on="timeseries-start" class="Bool (strict)"("Value"=FALSE ("timeseries-start")) -> ()  [unwired: 2 in, 2 out]
          }
        }
        n367 = Bundle("timeseries-current_image"=w398, "scan_image"=w400, "timeseries-start"=w401, "timeseries-next_scan"=w399, "timeseries-rem_time"=w397) -> (w402:T35)  [unwired: 1 in]
        n368 = call-by-ref "Start Asynchronous Call"(reference=w395, error in=w396, "period_s"="timeseries-period", "pixel_dwell_ms"=w418, "timeseries-autofocus"="timeseries-autofocus", "date_stop"="timeseries-stopdate", "pos_start_xyz"=w415, "image_size_x_um"=w414, "frame_size_x_px"=w413, "pos_start"=w412, "scan_direction"=w411, "GUI_references"=w402, "z-stack_parameters"=w405) -> ()  [unwired: 4 in, 3 out]
      }
      frame "saveImage" {
        w468 = T29 {"file_path"=path "", "file_name"="", "image"=[], "image_size_xy"={"image_size_x_um"=1.0, "image_size_y_um"=1.0}, "pixel_dwell_time_ms"=1.0, "Laser_power_mW"=1.0, "pixel_size"=0.0, "tile_ij"={"tile_i"=0, "tile_j"=0}, "Objective"="", "ColorMarkers"=[], "timestamp"=timestamp(0 s since 1904-01-01), "micro-position-xyz"={"micro-position_x_mm"=1.0, "micro-position_y_mm"=1.0, "micro-position_z_mm"=1.0}, "zero_xyz"={"zero_x_mm"=0.0, "zero_y_mm"=0.0, "zero_z_mm"=0.0}, "nano-position-xyz"={"nano-position_x_V"=1.0, "nano-position_y_V"=1.0, "nano-position_z_V"=1.0}, "Kxyz"={"Kx_V/um"=1.0, "Ky_V/um"=1.0, "Kz_V/um"=1.0}}  # image_info
        n369 = Bundle("pos-start_x"=w444, "pos-start_y"=w443, "focus_z"=w434) -> (w442:T28)  [unwired: 1 in]
        n370 = property class="IntGraph (strict)"(reference=w455) -> ("ZScale.MarkerVals[]"=w454:cluster{dbl, u32}[])  [unwired: 1 in, 2 out]
        n371 = property on="upos-x" class="DigNum (strict)"() -> ("Value"=w452:dbl)  [unwired: 2 in, 2 out]
        n372 = property on="upos-y" class="DigNum (strict)"() -> ("Value"=w451:dbl)  [unwired: 2 in, 2 out]
        n373 = property on="Laser power [mW]" class="DigNum (strict)"() -> ("Value"=w460:dbl)  [unwired: 2 in, 2 out]
        n374 = property on="pixel_size_x_um" class="DigNum (strict)"() -> ("Value"=w459:dbl)  [unwired: 2 in, 2 out]
        n375 = property on="objective" class="Ring (strict)"() -> ("Strings []"=w458:string[])  [unwired: 2 in, 2 out]
        n376 = property on="objective" class="Ring (strict)"() -> ("Value"=w457:u16)  [unwired: 2 in, 2 out]
        n377 = global read "GLOBAL_VAR.vi" "Ky"() -> (w440:dbl)
        n378 = global read "GLOBAL_VAR.vi" "Kx"() -> (w441:dbl)
        n379 = global read "GLOBAL_VAR.vi" "Kz"() -> (w439:dbl)
        n380 = Get Date/Time In Seconds() -> (seconds since 1Jan1904=w453:timestamp)
        n381 = Bundle("Value"=w452, "Value"=w451, "upos-y"=0.0) -> (w449:cluster{"Value":dbl, "Value":dbl, "upos-y":dbl})  [unwired: 1 in]
        n382 = Bundle("X Zero"=w447, "Y Zero"=w446, "upos-y"=0.0) -> (w445:T36)  [unwired: 1 in]
        n383 = Index Array(array=w458, index=w457) -> (element=w456:string)
        n384 = Bundle("Kx"=w441, "Ky"=w440, "Kz"=w439) -> (w438:cluster{"Kx":dbl, "Ky":dbl, "Kz":dbl})  [unwired: 1 in]
        n385 = Bundle("image_size_x_um"=w462, "image_size_x_um"=w462) -> (w463:T30)  [unwired: 1 in]
        n386 = Bundle By Name(cluster=w468, "file_path"=w466, "file_name"=w465, "image"=w464, "image_size_xy"=w463, "pixel_dwell_time_ms"=w461, "Laser_power_mW"=w460, "pixel_size"=w459, "Objective"=w456, "ColorMarkers"=w454, "timestamp"=w453, "micro-position-xyz"=w449, "zero_xyz"=w445, "nano-position-xyz"=w442, "Kxyz"=w438) -> (w467:T29)
        n387 = call "saveImage.vi"("save_txt"="save_txt", "save_tiff"="save_tiff", "image_info"=w467) -> ()  [unwired: 9 in]
      }
      frame "doT1" {
        n388 = property on="scan_image" class="IntGraph (strict)"() -> ("Cursor.Cursor X"=w474:dbl, "Cursor.Cursor Y"=w473:dbl)  [unwired: 2 in, 2 out]
        n389 = Bundle By Name(cluster=T11 {"nano-position_X_um"=0.0, "nano-position_Y_um"=0.0, "nano-position Z_um"=0.0} ("input_xyz"), "nano-position_X_um"=w474, "nano-position_Y_um"=w473, "nano-position Z_um"=w471) -> (w472:T11)
        n390 = flat-sequence {
          tunnel: path "C:/SpinCore/SpinAPI/dll/spinapi64.dll" ("path in") -> [w485]
          tunnel: [w484] -> w482
          tunnel: [w483] -> w481
          tunnel: w482 -> [_]
          tunnel: w481 -> [_]
          tunnel: w472 -> [w487]
          frame #0 {
            n391 = call "pb-stop.vi"("path in"=w485) -> ("error out"=w483:errorcluster, "path out"=w484:path)  [unwired: 9 in]
            n392 = Wait (ms)(milliseconds to wait=u32 100) -> ()  [unwired: 1 out]
          }
          frame #1 {
            n393 = call "gui_T1.vi"("input_xyz"=w487) -> ()  [unwired: 11 in]
            n394 = property on="laser_on-off" class="Bool (strict)"("Value"=FALSE ("laser_on-off")) -> ()  [unwired: 2 in, 2 out]
          }
        }
      }
      frame "doRecenter" {
        n395 = while {
          stop <- w494 continue-if-true
          n396 = property on="scan_image" class="IntGraph (strict)"() -> ("Cursor.Cursor X"=w506:dbl, "Cursor.Cursor Y"=w505:dbl)  [unwired: 2 in, 2 out]
          n397 = property on="focus_z" class="DigNum (strict)"() -> ("Value"=w504:dbl)  [unwired: 2 in, 2 out]
          n398 = Bundle("Cursor.Cursor X"=w506, "Cursor.Cursor Y"=w505, "Value"=w504) -> (w503:T37)  [unwired: 1 in]
          n399 = call "center_particle.vi"("input_xyz"=w503, "parameters_xy-scan"="parameters_xy-scan", "parameters_z-scan"="parameters_z-scan") -> ("output_xyz"=w500:T11, "particle_lost"=w496:bool)  [unwired: 9 in, 2 out]
          "particle_lost" <- w496
          n400 = Not(x=w496) -> (.not. x?=w493:bool)
          n401 = Unbundle By Name(w500) -> ("nano-position_X_um"=w498:sgl, "nano-position_Y_um"=w497:sgl, "nano-position Z_um"=w499:sgl)
          n402 = property on="scan_image" class="IntGraph (strict)"("Cursor.Cursor X"=w498, "Cursor.Cursor Y"=w497) -> ()  [unwired: 2 in, 2 out]
          n403 = property on="focus_z" class="DigNum (strict)"("Value"=w499) -> ()  [unwired: 2 in, 2 out]
          n404 = And(x="continious_recenter", y=w493) -> (x .and. y?=w494:bool)
        }
      }
    }
  }
  n405 = Unregister For Events(event registration refnum=w21) -> (error out=w20:errorcluster)  [unwired: 1 in]
  n406 = Destroy User Event(user event=w15, error in=w20) -> ()  [unwired: 1 out]
  n407 = Release Queue(queue=w19) -> ()  [unwired: 2 in, 3 out]
  n408 = call <instrlib>:"PM100D Close.vi"("error in (no error)"=w9, "instrument handle"=w8) -> ()  [unwired: 9 in, 1 out]
